vi "Phase III control screen.vi"() -> ()   [LabVIEW 2020]
uses:
  UI Message handler/User Event - Stop/User Event - Stop.lvlib
  UI Message handler/Message Queue/Message Queue.lvlib
  Globals/Phase III Globals.vi
  Controls/boolean ref.ctl
  Controls/Config.ctl
panel:
  out "Decerleration- LOX":bool
  out "Steady- LOX":bool
  out "Acceleration LOX":bool
  in  "Exit RT":bool
  in  "Check Prefire Purge Preparation Readiness 19":bool
  in  "Check Prefire Purge Preparation Readiness 18":bool
  in  "Check Prefire Purge Preparation Readiness 17":bool
  in  "Check Prefire Purge Preparation Readiness 16":bool
  in  "Check Prefire Purge Preparation Readiness 15":bool
  in  "Check Prefire Purge Preparation Readiness 14":bool
  in  "Check Prefire Purge Preparation Readiness 13":bool
  in  "Check Prefire Purge Preparation Readiness 12":bool
  in  "Check Prefire Purge Preparation Readiness 11":bool
  in  "Check Prefire Purge Preparation Readiness 10":bool
  in  "Check Prefire Purge Preparation Readiness 9":bool
  in  "Check Prefire Purge Preparation Readiness 8":bool
  in  "Check Prefire Purge Preparation Readiness 7":bool
  in  "Check Prefire Purge Preparation Readiness 6":bool
  out "PPSU":bool
  out "RUN ACKNOWLEDGE LOX":bool
  out "Shaft Rotational Direction":string
  out "Speed RPM -lox":dbl format="%#_g r/min"
  out "Frequency":dbl format="%#_g Hz"
  in  "SPEED                      l":dbl format="%#_g r/m"
  in  "RAMP DOWN      l":dbl format="%#_g S"
  in  "RAMP UP             l":dbl format="%#_g S"
  in  "SET FREQ             l":dbl format="%#_g Hz"
  out "RUN ACKNOWLEDGE Atf":bool
  out "Shaft Rotational Direction":string
  out "Speed RPM":dbl format="%#_g r/min"
  out "Frequency":dbl format="%#_g Hz"
  out "Terminal Power":dbl format="%#_g W"
  out "Terminal Current":dbl format="%#_g A"
  out "Terminal Voltage":dbl format="%#_g V"
  out "C_EPV_16 HSS":bool
  in  "C_EPV_16":bool
  out "N_EPV_202 HSS":bool
  in  "N_EPV_202":bool
  out "C_EPV_1352 HSS":bool
  in  "C_EPV_1352":bool
  out "C_EPV_18 HSS":bool
  in  "C_EPV_18":bool
  out "C_EPV_803 HSS":bool
  in  "C_EPV_803":bool
  out "N_EPV_141 HSS":bool
  in  "N_EPV_141":bool
  out "G_EPV_51 HSS":bool
  in  "G_EPV_51":bool
  out "N_EPV_61 HSS":bool
  in  "N_EPV_61":bool
  out "N_EPV_62b HSS":bool
  in  "N_EPV_62b":bool
  out "N_EPV_62a HSS":bool
  in  "N_EPV_62a":bool
  out "C_EPV_127 HSS":bool
  in  "C_EPV_127":bool
  out "C_EPV_123 HSS":bool
  in  "C_EPV_123":bool
  out "C_EPV_8 HSS":bool
  in  "C_EPV_8":bool
  out "C_EPV_7 HSS":bool
  in  "C_EPV_7":bool
  out "C_EPV_2 HSS":bool
  in  "C_EPV_2":bool
  out "N_EPV_75 HSS":bool
  in  "F_EPV_75":bool
  out "N_EPV_206 HSS":bool
  in  "N_EPV_206":bool
  out "N_EPV_203 HSS":bool
  in  "N_EPV_203":bool
  out "F_EPV_28 HSS":bool
  in  "F_EPV_28":bool
  out "N_EPV_142 HSS":bool
  in  "F_EPV_142":bool
  out "N_EPV_33 HSS":bool
  in  "N_EPV_ 33":bool
  out "N_EPV_69 HSS":bool
  in  "N_EPV_ 69":bool
  out "N_EPV_68 HSS":bool
  in  "N_EPV_68":bool
  out "F_EPV_41 HSS":bool
  in  "F_EPV_41":bool
  out "F_EPV_21 HSS":bool
  in  "F_EPV_21":bool
  out "F_EPV_132 HSS":bool
  in  "F_EPV_132":bool
  out "F_EPV_131 HSS":bool
  in  "F_EPV_131":bool
  out "F_EPV_136 HSS":bool
  in  "F_EPV_136":bool
  out "MS failure":bool
  out "Over power detection":bool
  out "Over current detection":bool
  out "over voltage detection":bool
  out "power failure status":bool
  out "Decerleration- ATF":bool
  out "Steady- ATF":bool
  out "Acceleration atf":bool
  out "LOG":bool
  out "TARGET":bool
  out "DR L":bool
  out "DR A":bool
  out "DO":bool
  out "DI":bool
  out "AO":bool
  out "AI":bool
  in  "ADC reset ATF":bool
  in  "MCU reset ATF":bool
  in  "Gate driver ATF":bool
  in  "Motor off ATF":bool
  in  "Motor On ATF":bool
  in  "Update drive ATF":bool
  in  "Adc reset lox":bool
  in  "MCU Reset -LOX":bool
  in  "Gate driver- LOX":bool
  in  "DC off":bool
  in  "DC on":bool
  in  "update ppsu":bool
  in  "Motor Off lox":bool
  in  "Motor On lox":bool
  in  "Update drive lox":bool
  in  "STOP LOG":bool
  in  "SPEED":dbl format="%#_g r/m"
  in  "RAMP DOWN":dbl format="%#_g S"
  in  "RAMP UP":dbl format="%#_g S"
  in  "SET FREQ":dbl format="%#_g Hz"
  in  "SET POWER":dbl format="%#_g W"
  in  "SET CURRENT":dbl format="%#_g A"
  in  "SET VOLTAGE":dbl format="%#_g V"
  in  "OPP(W)":dbl format="%#_g W"
  in  "OCP(A)":dbl format="%#_g A"
  in  "OVP(V)":dbl format="%#_g V"
  in  "Ms initialize":bool
  in  "Alarm ack":bool
  in  "Connect Drive Lox":bool
  in  "Connect Drive ATF":bool
  out "Time Stamp":timestamp format="%<%.3X>T"
  in  "Configure IP":bool
  in  "Datalog phase code":string(combo)
  in  "ABORT":bool
  in  "CONFIGURATION FILE":string(combo)
  in  "IP ADDRESS":string
  in  "HOLD UPDATE":bool
  in  "DAQ SETTING":bool
  in  "Connect ppsu":bool
  in  "Connect RT":bool
  in  "STOP DAQ":bool
  in  "EXIT":bool
  in  "START LOG":bool
  in  "START DAQ":bool
  # "VERSION NUMBER : 1.1"
  # "PHASE III"
  # "RELEASE DATE :03/05/24"
  # "Select the configuration file"
  # "Select the phase code"
  # "USER NAME :"
  # "SEQUENCE"
  # "ATF"
  # "LOX"
  # "ENGINE"
  # "EPV CONTROLS"
  # "EPV CONTROLS"
  # "EPV CONTROLS"
  # "Drive ATF Controls"
  # "Drive LOX Controls"
  # "PPSU"
  # "DRIVE ATF"
  # "DRIVE LOX"
  # "PPSU Controls"
  # "PPSU FEEDBACK PARAMETER"
  # "DRIVE ATF SET PARAMETER"
  # "Motor Rotational State"
  # "PPSU SET PARAMETER"
  # "DRIVE LOX SET PARAMETER"
  # "Motor Rotational State"
  # "PPSU FEEDBACK PARAMETER"
  # "DRIVE ATF FEEDBACK PARAMETER"
  # "DRIVE ATF FEEDBACK PARAMETER"
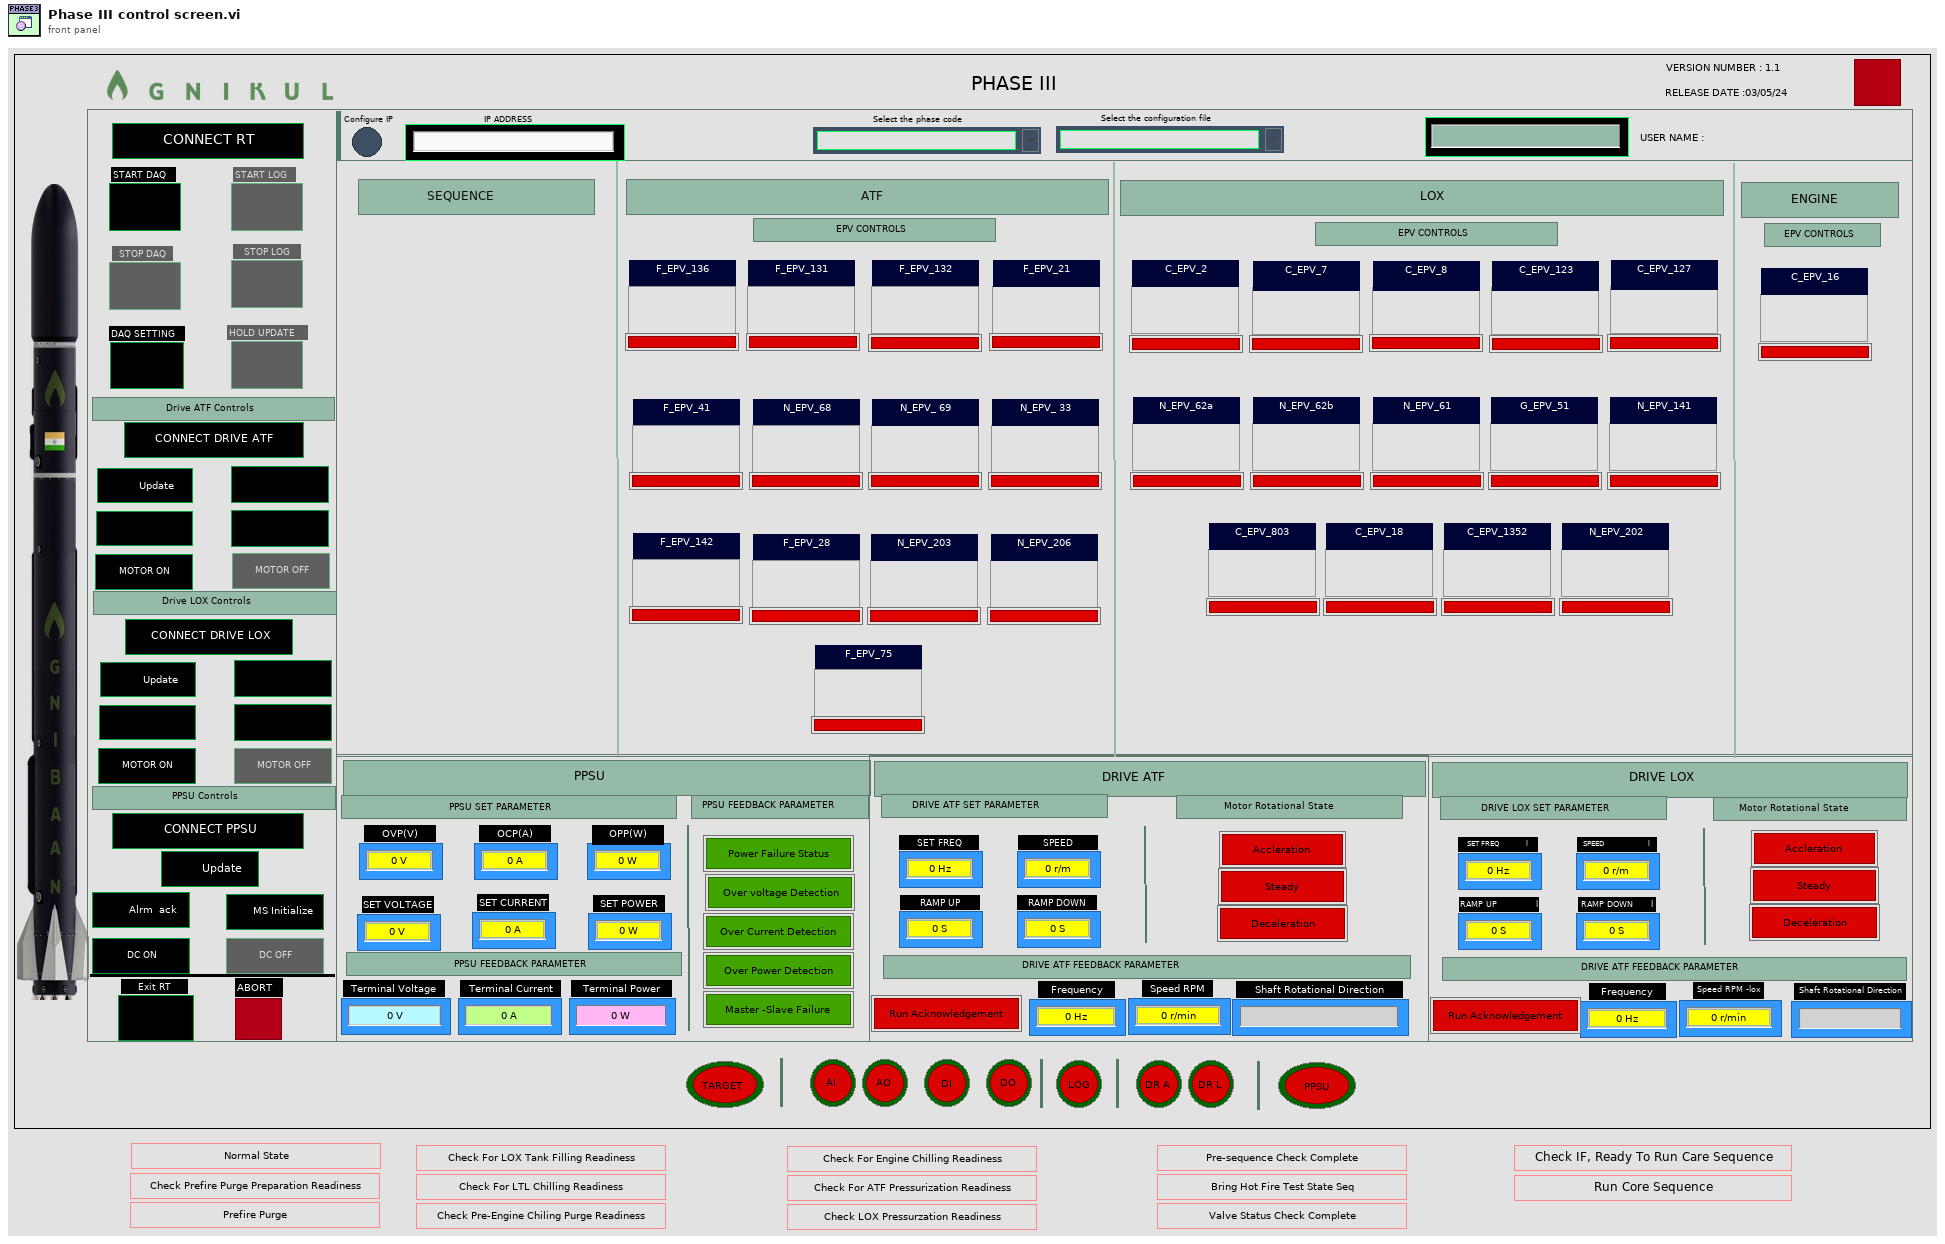
[diagram p1: front panel]
types:
  T1 = typedef "boolean ref.ctl" = cluster{"Connect RT":refnum<vi>, "START DAQ":refnum<vi>, "STOP DAQ":refnum<vi>, "DAQ SETTING":refnum<vi>, "START LOG":refnum<vi>, "STOP LOG":refnum<vi>, "Connect Drive ATF":refnum<vi>, "Update drive ATF":refnum<vi>, "Gate driver ATF":refnum<vi>, "Motor On ATF":refnum<vi>, "ADC reset ATF":refnum<vi>, "Gate driver ATF 2":refnum<vi>, "Motor off ATF":refnum<vi>, "MCU reset ATF":refnum<vi>, "Connect Drive Lox":refnum<vi>, "Update drive lox":refnum<vi>, "Gate driver- LOX":refnum<vi>, "Motor On lox":refnum<vi>, "Adc reset lox":refnum<vi>, "MCU Reset -LOX":refnum<vi>, "Motor Off lox":refnum<vi>, "Connect ppsu":refnum<vi>, "update ppsu":refnum<vi>, "DC on":refnum<vi>, "Alarm ack":refnum<vi>, "DC off":refnum<vi>, "Ms initialize":refnum<vi>, "Exit RT":refnum<vi>, "ABORT":refnum<vi>, "HOLD UPDATE":refnum<vi>}
  T2 = enum8{"Enabled", "Disabled", "Disabled and Grayed Out"}[]
  T3 = typedef "file folder ctl.ctl" = cluster{"Datalog path":path, "Configuration path":path, "Signal list path":path, "Sub vi's":path, "Authentication":path}
  T4 = typedef "Notifier ctl.ctl" = cluster{"Data":refnum<notifier>}
  T5 = typedef "Message Queue.lvlib/All Message Queues.ctl" = cluster{"UI":refnum<queue>, "NS ":refnum<queue>}
  T6 = typedef "Config.ctl" = cluster{"AO config":cluster{"Channel_Name":string, "Channel_Number":string, "Default_Value":dbl, "Units":string}[], "AI config":cluster{"Channel_Name":string, "Channel_Number":string, "Pre_Scale_min":dbl, "Pre_Scale_max":dbl, "Sensor_min":dbl, "Sensor_max":dbl, "Units":string}[], "DI config":cluster{"Channel_Name":string, "Channel_Number":string, "Default_Value":bool, "DI invert?":bool}[], "DO config":cluster{"Channel_Name":string, "Channel_Number":string, "Default_Value":bool, "DO invert?":bool}[], "TC config":cluster{"Channel_Name":string, "Channel_Number":string, "Pre_Scale_min":dbl, "Pre_Scale_max":dbl, "units":i32, " type":i32}[], "ACC config":cluster{"Channel_Name":string, "Channel_Number":string, "Pre_Scale_min":dbl, "Pre_Scale_max":dbl, "Terminal configuration":i32, "Sensitivity":dbl, "Sensitivity units":i32}[], "SG config":cluster{"Channel_Name":string, "Channel_Number":string, "Pre_Scale_min":dbl, "Pre_Scale_max":dbl}[], "Strain Gauge Settings":cluster{"poisson ratio":dbl, "nominal gage resistance":dbl, "gage factor":dbl}, "Bridge Settings":cluster{"voltage excitation value":dbl, "voltage excitation source":i32, "initial bridge voltage":dbl, "lead wire resistance":dbl, "strain configuration":i32}, "Sample Rate":cluster{"AI Sample Rate":dbl[], "AO Sample Rate":dbl[], "DI Sample Rate":dbl[], "TC Sample Rate":dbl[], "DO Sample Rate":dbl[], "SG Sample Rate":dbl[], "ACC Sample Rate":dbl[]}}
  T7 = enum16{"open", "replace", "create", "open or create", "replace or create", "replace or create with confirmation"}
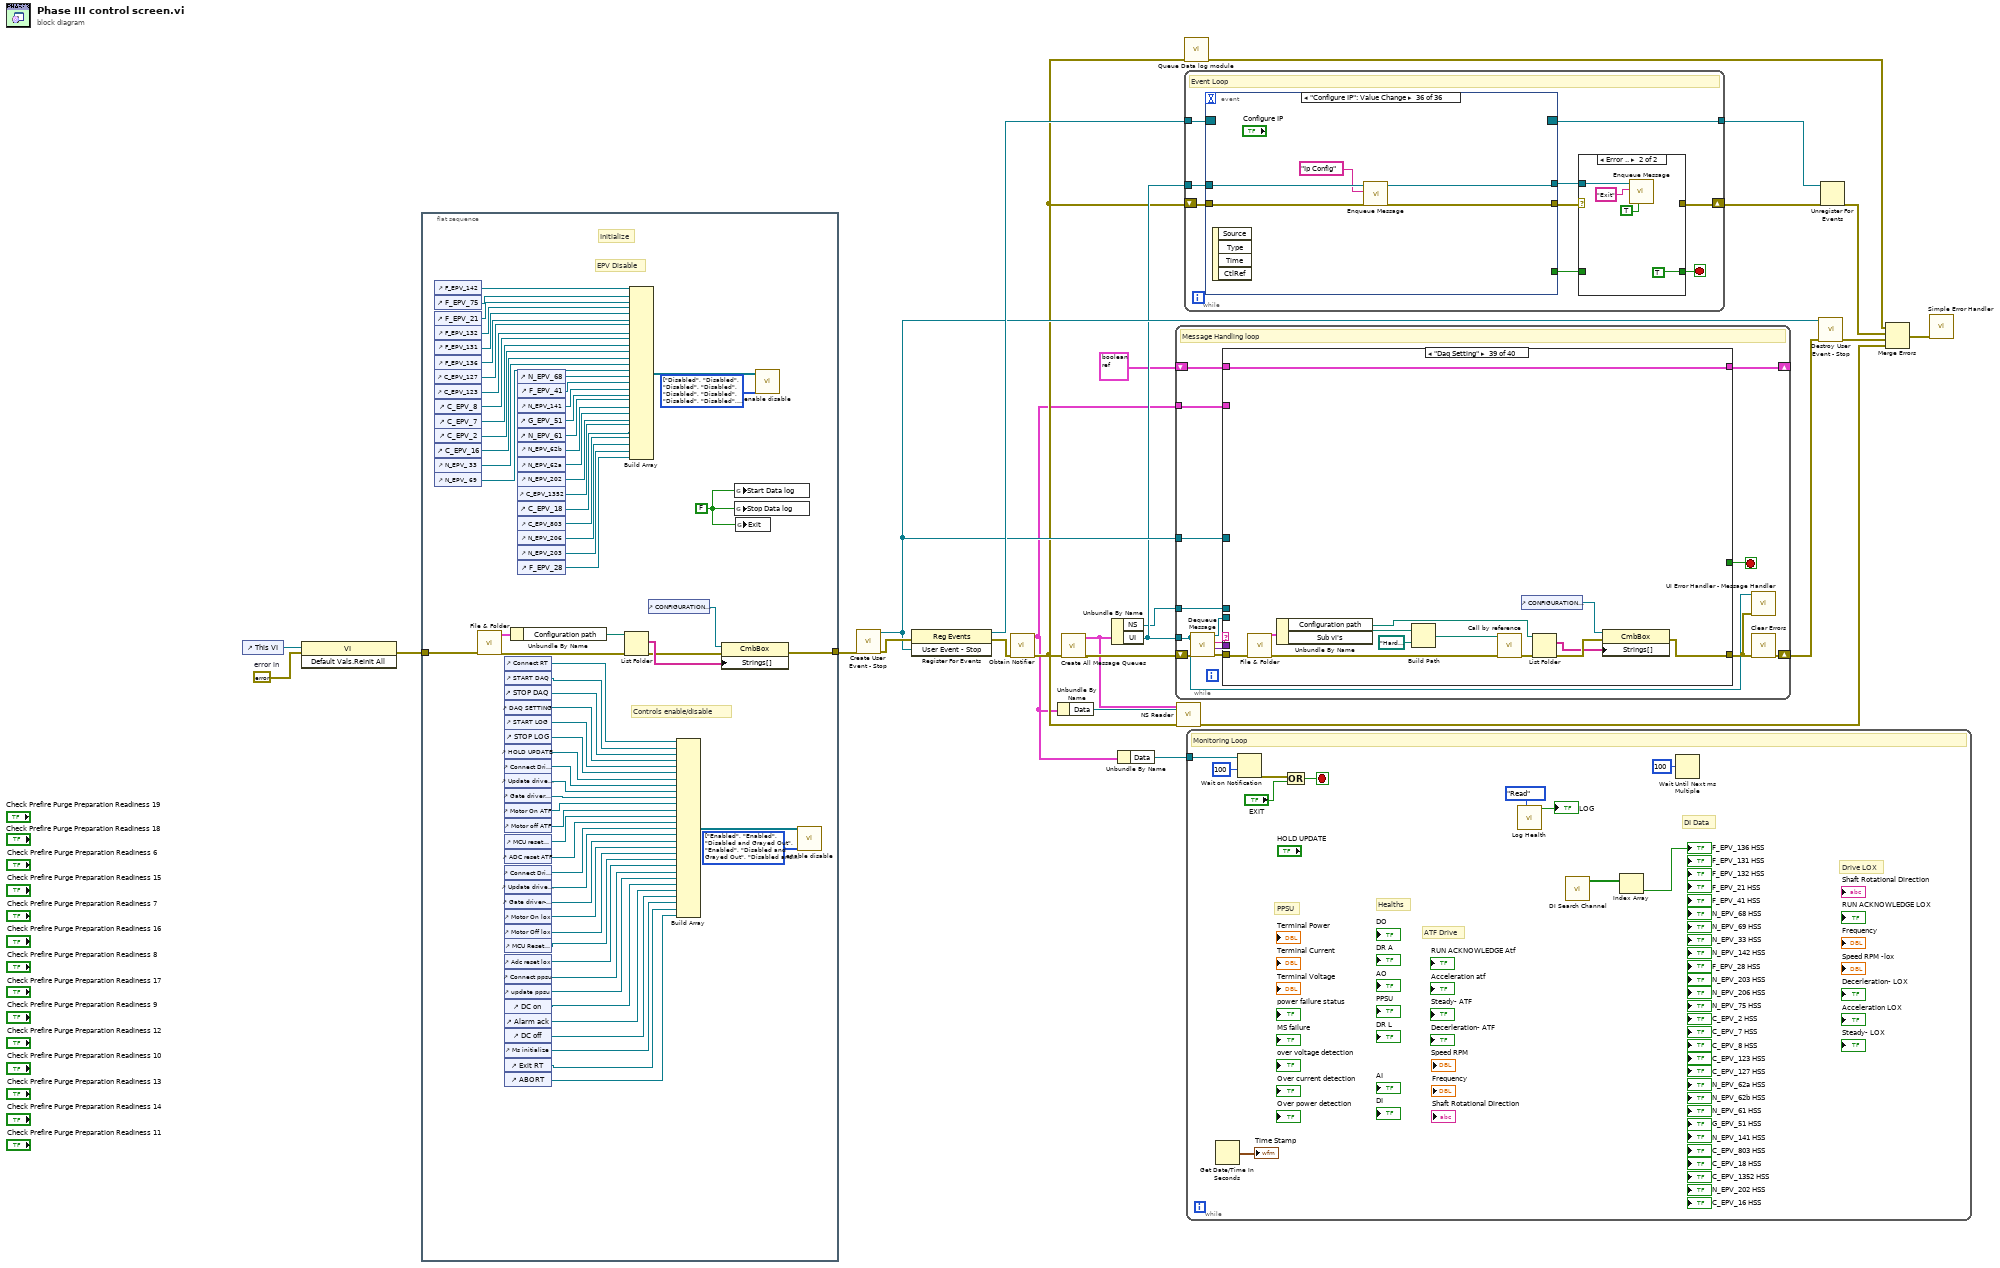
[diagram p0: block diagram]
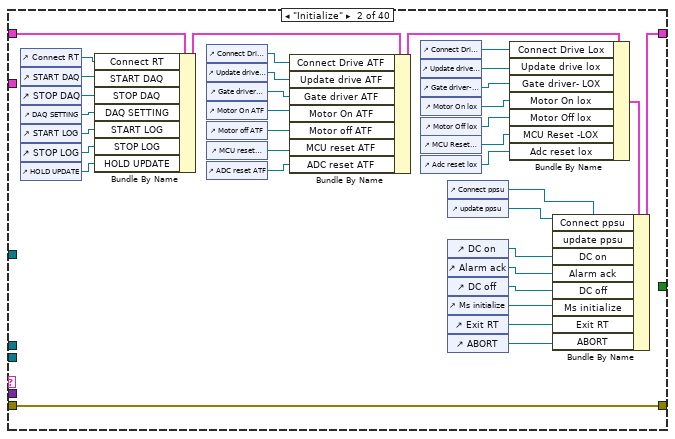
[diagram p3: hidden frame]
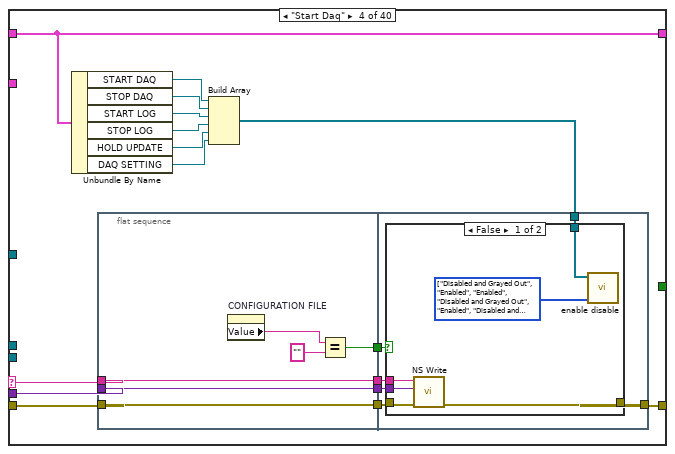
[diagram p5: hidden frame]
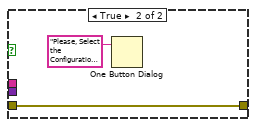
[diagram p6: hidden frame]
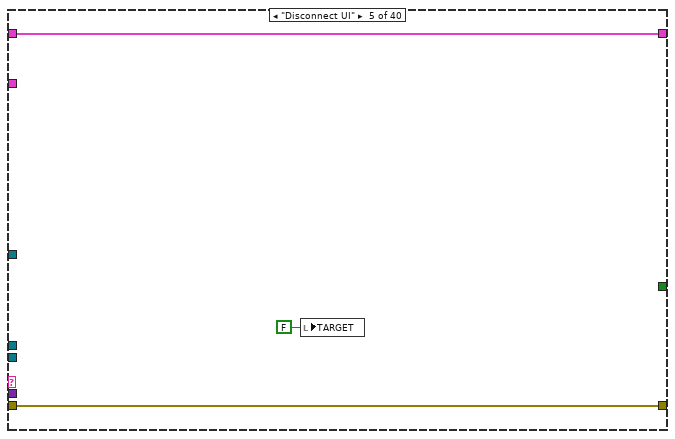
[diagram p7: hidden frame]
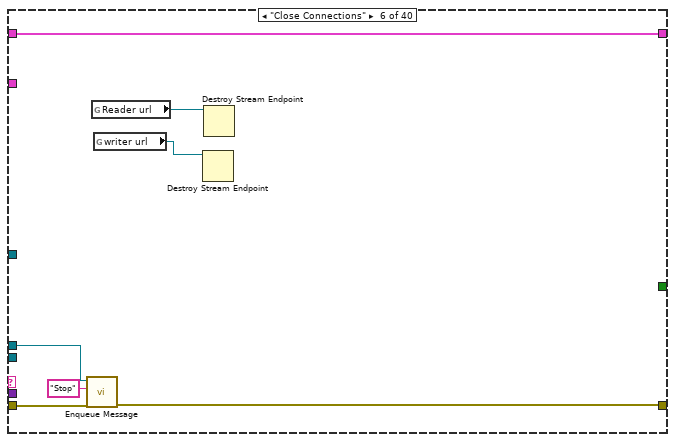
[diagram p8: hidden frame]
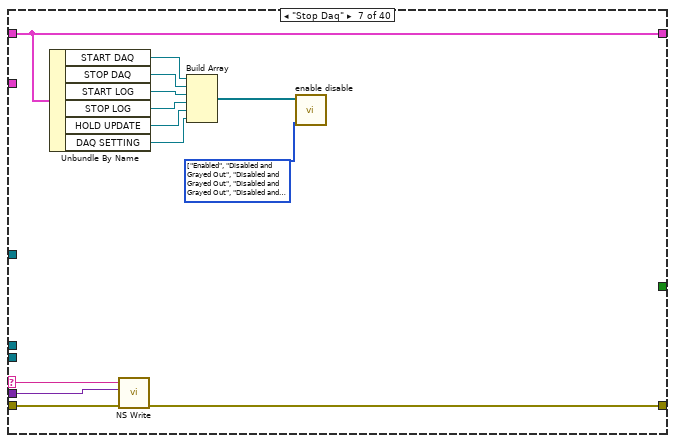
[diagram p9: hidden frame]
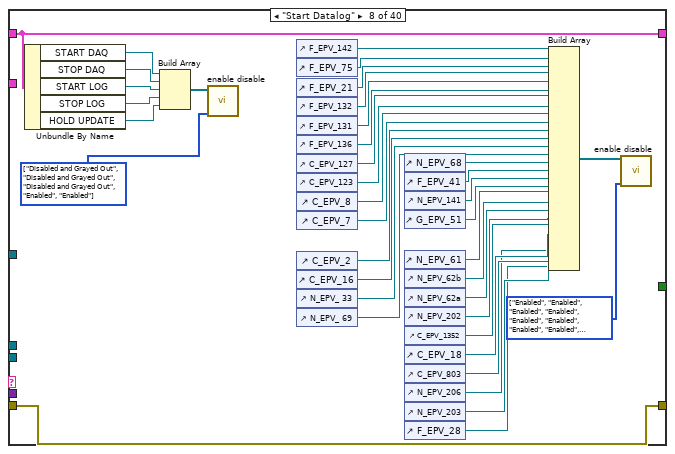
[diagram p10: hidden frame]
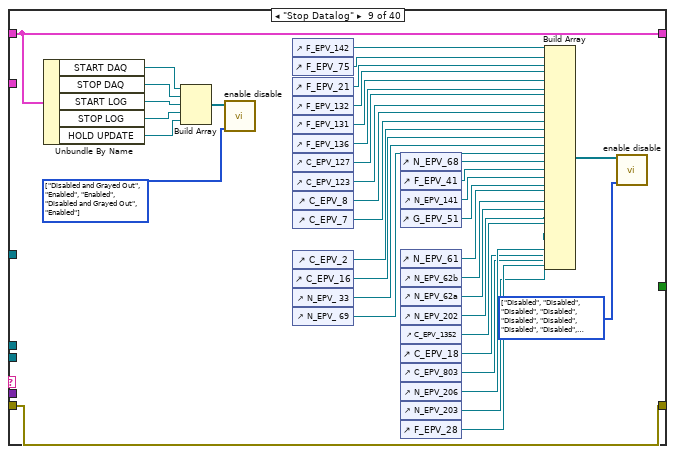
[diagram p11: hidden frame]
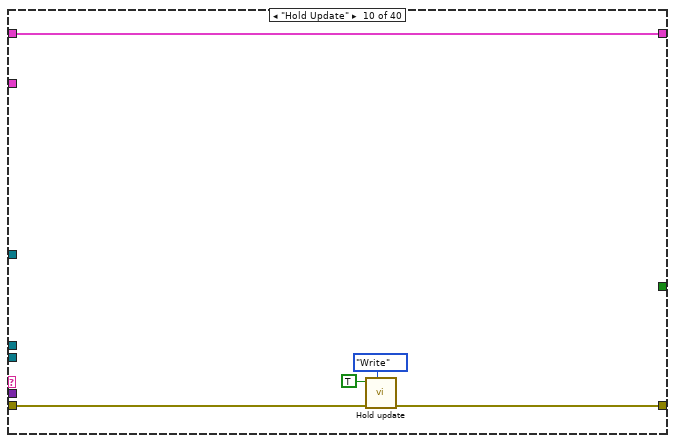
[diagram p12: hidden frame]
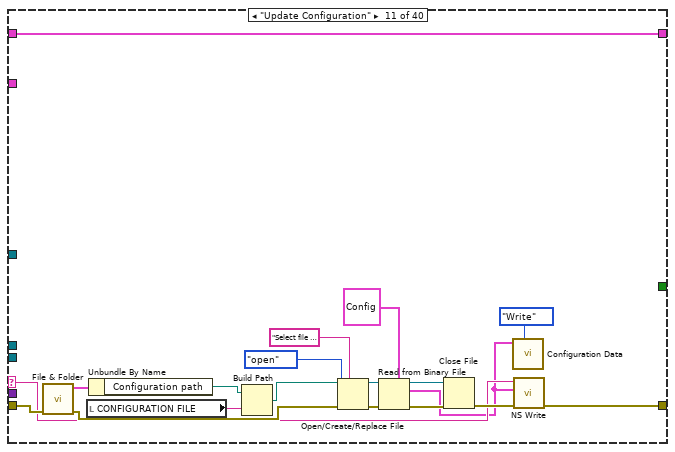
[diagram p13: hidden frame]
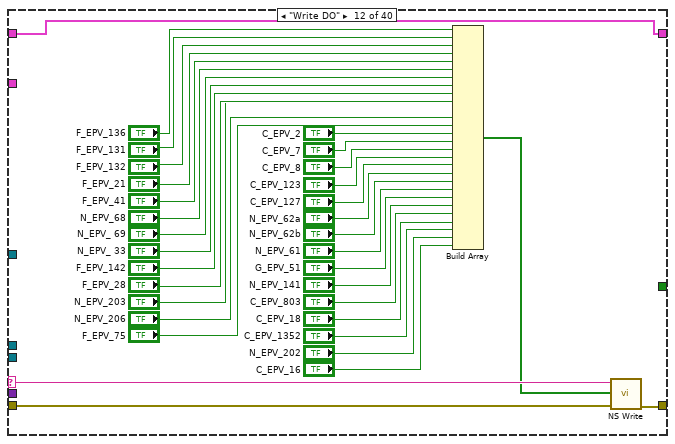
[diagram p14: hidden frame]
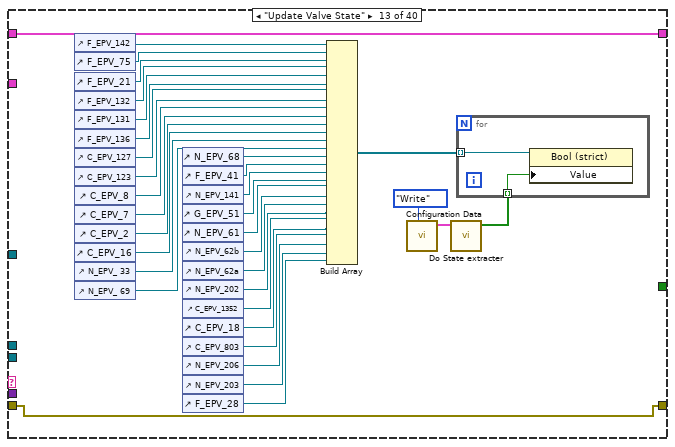
[diagram p15: hidden frame]
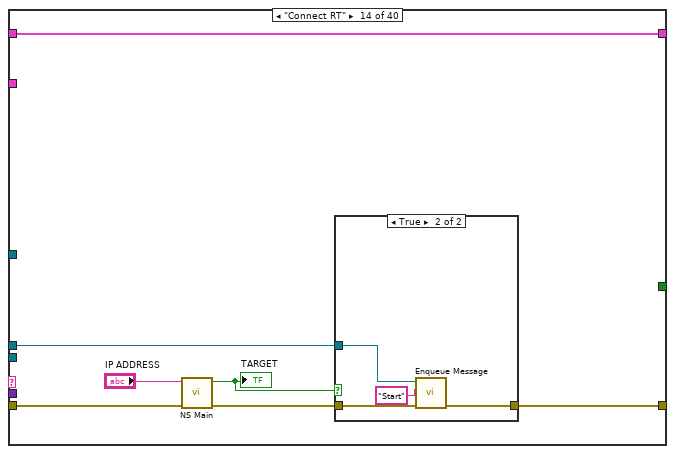
[diagram p16: hidden frame]
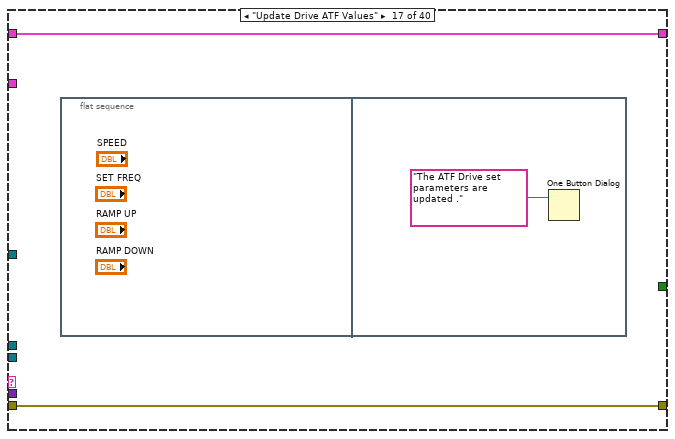
[diagram p20: hidden frame]
diagram:
  w2 = errorcluster {"status"=FALSE, "code"=0, "source"=""}  # error in
  n1 = control-ref of="This VI"() -> (w4:refnum<vi>)
  n2 = invoke class="VI" method="Default Vals.Reinit All"(reference=w4, error in=w2) -> (error out=w1:errorcluster)  [unwired: 1 in, 2 out]
  n3 = flat-sequence {
    tunnel: w1 -> [w31]
    tunnel: [w33] -> w16
    frame #0 {
      w34 = T2 [enum."Disabled", enum."Disabled", enum."Disabled", enum."Disabled", enum."Disabled", enum."Disabled", enum."Disabled", enum."Disabled", enum."Disabled", enum."Disabled", enum."Disabled", enum."Disabled", enum."Disabled", enum."Disabled", enum."Disabled", enum."Disabled", enum."Disabled", enum."Disabled", enum."Disabled", enum."Disabled", enum."Disabled", enum."Disabled", enum."Disabled", enum."Disabled", enum."Disabled", enum."Disabled", enum."Disabled", enum."Enabled", enum."Disabled"] items=["Enabled", "Disabled", "Disabled and Grayed Out"] ("Disabled")
      w65 = T2 [enum."Enabled", enum."Enabled", enum."Disabled and Grayed Out", enum."Enabled", enum."Disabled and Grayed Out", enum."Disabled and Grayed Out", enum."Disabled and Grayed Out", enum."Enabled", enum."Enabled", enum."Enabled", enum."Enabled", enum."Disabled and Grayed Out", enum."Enabled", enum."Enabled", enum."Enabled", enum."Enabled", enum."Enabled", enum."Enabled", enum."Disabled and Grayed Out", enum."Enabled", enum."Enabled", enum."Enabled", enum."Enabled", enum."Enabled", enum."Enabled", enum."Disabled and Grayed Out", enum."Enabled", enum."Enabled", enum."Enabled"] items=["Enabled", "Disabled", "Disabled and Grayed Out"] ("Disabled")
      w95 = FALSE ("Start Data log")
      # "Controls enable/disable"
      # "EPV Disable"
      # "Initialize"
      n4 = control-ref of="F_EPV_142"() -> (w35:refnum<vi>)
      n5 = control-ref of="F_EPV_75"() -> (w36:refnum<vi>)
      n6 = control-ref of="F_EPV_21"() -> (w37:refnum<vi>)
      n7 = control-ref of="F_EPV_132"() -> (w38:refnum<vi>)
      n8 = control-ref of="F_EPV_131"() -> (w39:refnum<vi>)
      n9 = control-ref of="F_EPV_136"() -> (w40:refnum<vi>)
      n10 = control-ref of="C_EPV_127"() -> (w41:refnum<vi>)
      n11 = control-ref of="C_EPV_123"() -> (w42:refnum<vi>)
      n12 = control-ref of="C_EPV_8"() -> (w43:refnum<vi>)
      n13 = control-ref of="C_EPV_7"() -> (w44:refnum<vi>)
      n14 = control-ref of="C_EPV_2"() -> (w45:refnum<vi>)
      n15 = control-ref of="C_EPV_16"() -> (w46:refnum<vi>)
      n16 = control-ref of="N_EPV_ 33"() -> (w47:refnum<vi>)
      n17 = control-ref of="N_EPV_ 69"() -> (w48:refnum<vi>)
      n18 = call "File & Folder.vi"("error in (no error)"=w31) -> ("error out"=w27:errorcluster, "File Output"=w30:T3)  [unwired: 9 in]
      n19 = control-ref of="Connect RT"() -> (w94:refnum<vi>)
      n20 = control-ref of="START DAQ"() -> (w93:refnum<vi>)
      n21 = control-ref of="STOP DAQ"() -> (w92:refnum<vi>)
      n22 = control-ref of="DAQ SETTING"() -> (w91:refnum<vi>)
      n23 = control-ref of="START LOG"() -> (w90:refnum<vi>)
      n24 = control-ref of="STOP LOG"() -> (w89:refnum<vi>)
      n25 = control-ref of="HOLD UPDATE"() -> (w88:refnum<vi>)
      n26 = control-ref of="Connect Drive ATF"() -> (w87:refnum<vi>)
      n27 = control-ref of="Update drive ATF"() -> (w86:refnum<vi>)
      n28 = control-ref of="Gate driver ATF"() -> (w85:refnum<vi>)
      n29 = control-ref of="Motor On ATF"() -> (w84:refnum<vi>)
      n30 = control-ref of="Motor off ATF"() -> (w83:refnum<vi>)
      n31 = control-ref of="MCU reset ATF"() -> (w82:refnum<vi>)
      n32 = control-ref of="ADC reset ATF"() -> (w81:refnum<vi>)
      n33 = control-ref of="Connect Drive Lox"() -> (w80:refnum<vi>)
      n34 = control-ref of="Update drive lox"() -> (w79:refnum<vi>)
      n35 = control-ref of="Gate driver- LOX"() -> (w78:refnum<vi>)
      n36 = control-ref of="Motor On lox"() -> (w77:refnum<vi>)
      n37 = control-ref of="Motor Off lox"() -> (w76:refnum<vi>)
      n38 = control-ref of="MCU Reset -LOX"() -> (w75:refnum<vi>)
      n39 = control-ref of="Adc reset lox"() -> (w74:refnum<vi>)
      n40 = control-ref of="Connect ppsu"() -> (w73:refnum<vi>)
      n41 = control-ref of="update ppsu"() -> (w72:refnum<vi>)
      n42 = control-ref of="DC on"() -> (w71:refnum<vi>)
      n43 = control-ref of="Alarm ack"() -> (w70:refnum<vi>)
      n44 = control-ref of="DC off"() -> (w69:refnum<vi>)
      n45 = control-ref of="Ms initialize"() -> (w68:refnum<vi>)
      n46 = control-ref of="Exit RT"() -> (w67:refnum<vi>)
      n47 = control-ref of="ABORT"() -> (w66:refnum<vi>)
      n48 = Unbundle By Name(w30) -> ("Configuration path"=w29:path)
      n49 = control-ref of="N_EPV_68"() -> (w49:refnum<vi>)
      n50 = control-ref of="F_EPV_41"() -> (w50:refnum<vi>)
      n51 = control-ref of="N_EPV_141"() -> (w51:refnum<vi>)
      n52 = control-ref of="G_EPV_51"() -> (w52:refnum<vi>)
      n53 = control-ref of="N_EPV_61"() -> (w53:refnum<vi>)
      n54 = control-ref of="N_EPV_62b"() -> (w54:refnum<vi>)
      n55 = control-ref of="N_EPV_62a"() -> (w55:refnum<vi>)
      n56 = control-ref of="N_EPV_202"() -> (w56:refnum<vi>)
      n57 = control-ref of="C_EPV_1352"() -> (w57:refnum<vi>)
      n58 = control-ref of="C_EPV_18"() -> (w58:refnum<vi>)
      n59 = control-ref of="C_EPV_803"() -> (w59:refnum<vi>)
      n60 = control-ref of="N_EPV_206"() -> (w60:refnum<vi>)
      n61 = control-ref of="N_EPV_203"() -> (w61:refnum<vi>)
      n62 = control-ref of="F_EPV_28"() -> (w62:refnum<vi>)
      n63 = List Folder(path=w29, error in=w27) -> (filenames=w28:string[], error out=w26:errorcluster)  [unwired: 2 in, 2 out]
      n64 = Build Array(w35, w36, w37, w38, w39, w40, w41, w42, w43, w44, w45, w46, w47, w48, w49, w50, w51, w52, w53, w54, w55, w56, w57, w58, w59, w60, w61, w62) -> (w63:refnum<vi>[])
      n65 = control-ref of="CONFIGURATION FILE"() -> (w32:refnum<vi>)
      n66 = Build Array(w94, w93, w92, w91, w90, w89, w88, w87, w86, w85, w84, w83, w82, w81, w80, w79, w78, w77, w76, w75, w74, w73, w72, w71, w70, w69, w68, w67, w66) -> (w64:refnum<vi>[])
      n67 = property class="CmbBox"(reference=w32, error in=w26, "Strings[]"=w28) -> (error out=w33:errorcluster)  [unwired: 1 out]
      n68 = global write "Phase III Globals.vi" "Start Data log"(w95) -> ()
      n69 = global write "Phase III Globals.vi" "Stop Data log"(w95) -> ()
      n70 = global write "Phase III Globals.vi" "Exit"(w95) -> ()
      n71 = call "enable disable.vi"("Disabled"=w34, "ref in"=w63) -> ()  [unwired: 10 in]
      n72 = call "enable disable.vi"("Disabled"=w65, "ref in"=w64) -> ()  [unwired: 10 in]
    }
  }
  n73 = call "Create User Event - Stop.vi"("error in (no error)"=w16) -> ("error out"=w22:errorcluster, "User Event - Stop"=w20:refnum<user-event>)  [unwired: 9 in]
  n74 = register-events(error in=w22, w20) -> (reference out=w25:refnum<event-registration>, error out=w15:errorcluster)  [unwired: 1 in]
  n75 = call "Obtain Notifier.vi"("error in"=w15) -> ("error out"=w8:errorcluster, "Notifier Out"=w5:T4)  [unwired: 9 in]
  n76 = Unbundle By Name(w5) -> ("Data"=w9:refnum<notifier>)
  n77 = call "Create All Message Queues.vi"("error in (no error)"=w8) -> ("error out"=w19:errorcluster, "Message Queues out"=w10:T5)  [unwired: 9 in]
  n78 = Unbundle By Name(w10) -> ("NS"=w6:refnum<queue>, "UI"=w18:refnum<queue>)
  n79 = Unbundle By Name(w5) -> ("Data"=w14:refnum<notifier>)
  n80 = while {
    shift-right: [w109] -> w13
    shift-left: w19 -> [w106]
    tunnel: w20 -> [w107]
    tunnel: w18 -> [w99]
    tunnel: w6 -> [w101]
    tunnel: w5 -> [w100]
    shift-right: [w96] -> _
    shift-left: T1 {"Connect RT"=refnum, "START DAQ"=refnum, "STOP DAQ"=refnum, "DAQ SETTING"=refnum, "START LOG"=refnum, "STOP LOG"=refnum, "Connect Drive ATF"=refnum, "Update drive ATF"=refnum, "Gate driver ATF"=refnum, "Motor On ATF"=refnum, "ADC reset ATF"=refnum, "Gate driver ATF 2"=refnum, "Motor off ATF"=refnum, "MCU reset ATF"=refnum, "Connect Drive Lox"=refnum, "Update drive lox"=refnum, "Gate driver- LOX"=refnum, "Motor On lox"=refnum, "Adc reset lox"=refnum, "MCU Reset -LOX"=refnum, "Motor Off lox"=refnum, "Connect ppsu"=refnum, "update ppsu"=refnum, "DC on"=refnum, "Alarm ack"=refnum, "DC off"=refnum, "Ms initialize"=refnum, "Exit RT"=refnum, "ABORT"=refnum, "HOLD UPDATE"=refnum} ("Cluster") -> [w97]
    stop <- w108 stop-if-true
    # "Message Handling loop"
    n81 = call "Dequeue Message.vi"("error in (no error)"=w106, "Message Queue"=w99) -> ("error out"=w105:errorcluster, "Message Data"=w102:variant, "Message"=w104:string, "dup Message Queue"=w103:refnum<queue>)  [unwired: 6 in]
    n82 = case shown="\"Daq Setting\"" w104 {
      selector: w104 -> [_ _ _ w163 _ _ w205 _ _ _ w293 w312 _ _ _ _ _ _ _ _ _ _ _ _ _ _ _ _ _ _ _ _ _ _ _ _ _ _ _ _]
      tunnel: w105 -> [w111 w146 w148 w162 w187 w190 w204 w208 w247 w289 w304 w314 w376 w385 w392 w394 w396 w399 w402 w404 w406 w416 w426 w428 w430 w432 w442 w452 w454 w463 w472 w474 w477 w479 w481 w486 w499 w504 w519 w521]
      tunnel: [w111 w146 w148 w161 w187 w188 w207 w208 w247 w288 w294 w313 w376 w380 w392 w394 w396 w399 w402 w404 w406 w416 w426 w428 w430 w432 w442 w452 w454 w463 w472 w474 w477 w479 w481 w493 w498 w502 w507 w521] -> w98
      tunnel: [_ _ _ _ _ _ _ _ _ _ _ _ _ _ _ _ _ _ _ _ _ _ _ _ _ _ _ _ _ _ _ _ _ _ _ TRUE ("EXIT") _ _ _ _] -> w108
      tunnel: w107 -> [_ _ _ _ _ _ _ _ _ _ _ _ _ _ _ _ _ _ _ _ _ _ _ _ _ _ _ _ _ _ _ _ _ _ _ w495 _ _ _ _]
      tunnel: w103 -> [_ _ _ _ _ _ _ _ _ _ _ _ _ _ _ _ _ _ _ _ _ _ _ _ _ _ _ _ _ _ _ _ _ _ _ w494 _ _ _ _]
      tunnel: w102 -> [_ _ _ w164 _ _ w206 _ _ _ _ _ _ _ _ _ _ _ _ _ _ _ _ _ _ _ _ _ _ _ _ _ _ _ _ _ _ _ _ _]
      tunnel: w101 -> [_ _ _ _ _ w189 _ _ _ _ _ _ _ w382 _ _ _ _ _ _ _ _ _ _ _ _ _ _ _ _ _ _ _ _ _ w484 _ _ _ _]
      tunnel: w100 -> [_ _ _ _ _ _ _ _ _ _ _ _ _ _ _ _ _ _ _ _ _ _ _ _ _ _ _ _ _ _ _ _ _ _ _ w491 _ _ _ _]
      tunnel: w97 -> [w110 w145 w147 w160 w185 w192 w196 w239 w279 w290 w309 w310 w375 w379 w391 w393 w395 w398 w401 w403 w405 w415 w418 w427 w429 w431 w441 w443 w453 w462 w464 w473 w476 w478 w480 w482 w501 w506 w513 w520]
      tunnel: [w110 w120 w147 w160 w185 w192 w196 w239 w279 w290 w309 w310 w375 w379 w391 w393 w395 w398 w401 w403 w405 w415 w418 w427 w429 w431 w441 w443 w453 w462 w464 w473 w476 w478 w480 w482 w501 w506 w513 w520] -> w96
      frame "Pole event", Default {
      }
      frame "Initialize" {
        n83 = control-ref of="Connect RT"() -> (w143:refnum<vi>)
        n84 = control-ref of="START DAQ"() -> (w142:refnum<vi>)
        n85 = control-ref of="STOP DAQ"() -> (w141:refnum<vi>)
        n86 = control-ref of="DAQ SETTING"() -> (w140:refnum<vi>)
        n87 = control-ref of="START LOG"() -> (w139:refnum<vi>)
        n88 = control-ref of="STOP LOG"() -> (w138:refnum<vi>)
        n89 = control-ref of="HOLD UPDATE"() -> (w137:refnum<vi>)
        n90 = Bundle By Name(cluster=w145, "Connect RT"=w143, "START DAQ"=w142, "STOP DAQ"=w141, "DAQ SETTING"=w140, "START LOG"=w139, "STOP LOG"=w138, "HOLD UPDATE"=w137) -> (w144:T1)
        n91 = control-ref of="Connect Drive ATF"() -> (w135:refnum<vi>)
        n92 = control-ref of="Update drive ATF"() -> (w134:refnum<vi>)
        n93 = control-ref of="Gate driver ATF"() -> (w133:refnum<vi>)
        n94 = control-ref of="Motor On ATF"() -> (w132:refnum<vi>)
        n95 = control-ref of="Motor off ATF"() -> (w131:refnum<vi>)
        n96 = control-ref of="MCU reset ATF"() -> (w130:refnum<vi>)
        n97 = control-ref of="ADC reset ATF"() -> (w129:refnum<vi>)
        n98 = Bundle By Name(cluster=w144, "Connect Drive ATF"=w135, "Update drive ATF"=w134, "Gate driver ATF"=w133, "Motor On ATF"=w132, "Motor off ATF"=w131, "MCU reset ATF"=w130, "ADC reset ATF"=w129) -> (w136:T1)
        n99 = control-ref of="Connect Drive Lox"() -> (w128:refnum<vi>)
        n100 = control-ref of="Update drive lox"() -> (w127:refnum<vi>)
        n101 = control-ref of="Gate driver- LOX"() -> (w126:refnum<vi>)
        n102 = control-ref of="Motor On lox"() -> (w125:refnum<vi>)
        n103 = control-ref of="Motor Off lox"() -> (w124:refnum<vi>)
        n104 = control-ref of="MCU Reset -LOX"() -> (w123:refnum<vi>)
        n105 = control-ref of="Adc reset lox"() -> (w122:refnum<vi>)
        n106 = control-ref of="Connect ppsu"() -> (w119:refnum<vi>)
        n107 = control-ref of="update ppsu"() -> (w118:refnum<vi>)
        n108 = control-ref of="DC on"() -> (w117:refnum<vi>)
        n109 = control-ref of="Alarm ack"() -> (w116:refnum<vi>)
        n110 = control-ref of="DC off"() -> (w115:refnum<vi>)
        n111 = control-ref of="Ms initialize"() -> (w114:refnum<vi>)
        n112 = control-ref of="Exit RT"() -> (w113:refnum<vi>)
        n113 = control-ref of="ABORT"() -> (w112:refnum<vi>)
        n114 = Bundle By Name(cluster=w136, "Connect Drive Lox"=w128, "Update drive lox"=w127, "Gate driver- LOX"=w126, "Motor On lox"=w125, "Motor Off lox"=w124, "MCU Reset -LOX"=w123, "Adc reset lox"=w122) -> (w121:T1)
        n115 = Bundle By Name(cluster=w121, "Connect ppsu"=w119, "update ppsu"=w118, "DC on"=w117, "Alarm ack"=w116, "DC off"=w115, "Ms initialize"=w114, "Exit RT"=w113, "ABORT"=w112) -> (w120:T1)
      }
      frame "Ip Config" {
      }
      frame "Start Daq" {
        n116 = Unbundle By Name(w160) -> ("START DAQ"=w159:refnum<vi>, "STOP DAQ"=w158:refnum<vi>, "START LOG"=w157:refnum<vi>, "STOP LOG"=w156:refnum<vi>, "HOLD UPDATE"=w155:refnum<vi>, "DAQ SETTING"=w154:refnum<vi>)
        n117 = flat-sequence {
          tunnel: w162 -> [w168]
          tunnel: w163 -> [w169]
          tunnel: w164 -> [w170]
          tunnel: [w170] -> w153
          tunnel: [w169] -> w152
          tunnel: [w168] -> w151
          tunnel: [w165] -> w150
          tunnel: [w173] -> w161
          tunnel: w153 -> [w176]
          tunnel: w152 -> [w175]
          tunnel: w151 -> [w174]
          tunnel: w150 -> [w172]
          tunnel: w149 -> [w171]
          frame #0 {
            n118 = property on="CONFIGURATION FILE" class="CmbBox"() -> ("Value"=w167:string)  [unwired: 2 in, 2 out]
            n119 = Equal?(x=w167, y="") -> (x = y?=w165:bool)
          }
          frame #1 {
            n120 = case shown="False" w172 {
              tunnel: w176 -> [w182 _]
              tunnel: w175 -> [w181 _]
              tunnel: w174 -> [w180 w184]
              tunnel: [w179 w184] -> w173
              tunnel: w171 -> [w178 _]
              frame False {
                w177 = T2 [enum."Disabled and Grayed Out", enum."Enabled", enum."Enabled", enum."Disabled and Grayed Out", enum."Enabled", enum."Disabled and Grayed Out"] items=["Enabled", "Disabled", "Disabled and Grayed Out"] ("Disabled")
                n121 = call "NS Write.vi"("error in"=w180, "Data"=w182, "Message"=w181) -> ("error out"=w179:errorcluster)  [unwired: 8 in]
                n122 = call "enable disable.vi"("Disabled"=w177, "ref in"=w178) -> ()  [unwired: 10 in]
              }
              frame True {
                n123 = One Button Dialog(message="Please, Select the Configuration File !!") -> ()  [unwired: 1 in, 1 out]
              }
            }
          }
        }
        n124 = Build Array(w159, w158, w157, w156, w155, w154) -> (w149:refnum<vi>[])
      }
      frame "Disconnect UI" {
        n125 = local write "TARGET"(FALSE ("TARGET")) -> ()
      }
      frame "Close Connections" {
        n126 = call "Enqueue Message.vi"("error in (no error)"=w190, "Message"="Stop", "Message Queue"=w189) -> ("error out"=w188:errorcluster)  [unwired: 7 in, 1 out]
        n127 = global read "Phase III Globals.vi" "Reader url"() -> (w194:refnum<k21>)
        n128 = global read "Phase III Globals.vi" "writer url"() -> (w193:refnum<k21>)
        n129 = Destroy Stream Endpoint(11:w193) -> ()  [unwired: 1 in, 1 out]
        n130 = Destroy Stream Endpoint(11:w194) -> ()  [unwired: 1 in, 1 out]
      }
      frame "Stop Daq" {
        w197 = T2 [enum."Enabled", enum."Disabled and Grayed Out", enum."Disabled and Grayed Out", enum."Disabled and Grayed Out", enum."Disabled and Grayed Out", enum."Enabled"] items=["Enabled", "Disabled", "Disabled and Grayed Out"] ("Disabled")
        n131 = Unbundle By Name(w196) -> ("START DAQ"=w203:refnum<vi>, "STOP DAQ"=w202:refnum<vi>, "START LOG"=w201:refnum<vi>, "STOP LOG"=w200:refnum<vi>, "HOLD UPDATE"=w198:refnum<vi>, "DAQ SETTING"=w195:refnum<vi>)
        n132 = call "NS Write.vi"("error in"=w204, "Data"=w206, "Message"=w205) -> ("error out"=w207:errorcluster)  [unwired: 8 in]
        n133 = Build Array(w203, w202, w201, w200, w198, w195) -> (w199:refnum<vi>[])
        n134 = call "enable disable.vi"("Disabled"=w197, "ref in"=w199) -> ()  [unwired: 10 in]
      }
      frame "Start Datalog" {
        w209 = T2 [enum."Enabled", enum."Enabled", enum."Enabled", enum."Enabled", enum."Enabled", enum."Enabled", enum."Enabled", enum."Enabled", enum."Enabled", enum."Enabled", enum."Enabled", enum."Enabled", enum."Enabled", enum."Enabled", enum."Enabled", enum."Enabled", enum."Enabled", enum."Enabled", enum."Enabled", enum."Enabled", enum."Enabled", enum."Enabled", enum."Enabled", enum."Enabled", enum."Enabled", enum."Enabled", enum."Enabled", enum."Enabled", enum."Enabled"] items=["Enabled", "Disabled", "Disabled and Grayed Out"] ("Disabled")
        w240 = T2 [enum."Disabled and Grayed Out", enum."Disabled and Grayed Out", enum."Disabled and Grayed Out", enum."Enabled", enum."Enabled"] items=["Enabled", "Disabled", "Disabled and Grayed Out"] ("Disabled")
        n135 = Unbundle By Name(w239) -> ("START DAQ"=w246:refnum<vi>, "STOP DAQ"=w245:refnum<vi>, "START LOG"=w244:refnum<vi>, "STOP LOG"=w243:refnum<vi>, "HOLD UPDATE"=w241:refnum<vi>)
        n136 = Build Array(w246, w245, w244, w243, w241) -> (w242:refnum<vi>[])
        n137 = call "enable disable.vi"("Disabled"=w240, "ref in"=w242) -> ()  [unwired: 10 in]
        n138 = control-ref of="F_EPV_142"() -> (w238:refnum<vi>)
        n139 = control-ref of="F_EPV_75"() -> (w237:refnum<vi>)
        n140 = control-ref of="F_EPV_21"() -> (w236:refnum<vi>)
        n141 = control-ref of="F_EPV_132"() -> (w235:refnum<vi>)
        n142 = control-ref of="F_EPV_131"() -> (w234:refnum<vi>)
        n143 = control-ref of="F_EPV_136"() -> (w233:refnum<vi>)
        n144 = control-ref of="C_EPV_127"() -> (w232:refnum<vi>)
        n145 = control-ref of="C_EPV_123"() -> (w231:refnum<vi>)
        n146 = control-ref of="C_EPV_8"() -> (w230:refnum<vi>)
        n147 = control-ref of="C_EPV_7"() -> (w229:refnum<vi>)
        n148 = control-ref of="C_EPV_2"() -> (w228:refnum<vi>)
        n149 = control-ref of="C_EPV_16"() -> (w227:refnum<vi>)
        n150 = control-ref of="N_EPV_ 33"() -> (w226:refnum<vi>)
        n151 = control-ref of="N_EPV_ 69"() -> (w225:refnum<vi>)
        n152 = control-ref of="N_EPV_68"() -> (w224:refnum<vi>)
        n153 = control-ref of="F_EPV_41"() -> (w223:refnum<vi>)
        n154 = control-ref of="N_EPV_141"() -> (w222:refnum<vi>)
        n155 = control-ref of="G_EPV_51"() -> (w221:refnum<vi>)
        n156 = control-ref of="N_EPV_61"() -> (w220:refnum<vi>)
        n157 = control-ref of="N_EPV_62b"() -> (w219:refnum<vi>)
        n158 = control-ref of="N_EPV_62a"() -> (w218:refnum<vi>)
        n159 = control-ref of="N_EPV_202"() -> (w217:refnum<vi>)
        n160 = control-ref of="C_EPV_1352"() -> (w216:refnum<vi>)
        n161 = control-ref of="C_EPV_18"() -> (w215:refnum<vi>)
        n162 = control-ref of="C_EPV_803"() -> (w214:refnum<vi>)
        n163 = control-ref of="N_EPV_206"() -> (w213:refnum<vi>)
        n164 = control-ref of="N_EPV_203"() -> (w212:refnum<vi>)
        n165 = control-ref of="F_EPV_28"() -> (w211:refnum<vi>)
        n166 = Build Array(w238, w237, w236, w235, w234, w233, w232, w231, w230, w229, w228, w227, w226, w225, w224, w223, w222, w221, w220, w219, w218, w217, w216, w215, w214, w213, w212, w211) -> (w210:refnum<vi>[])
        n167 = call "enable disable.vi"("Disabled"=w209, "ref in"=w210) -> ()  [unwired: 10 in]
      }
      frame "Stop Datalog" {
        w248 = T2 [enum."Disabled", enum."Disabled", enum."Disabled", enum."Disabled", enum."Disabled", enum."Disabled", enum."Disabled", enum."Disabled", enum."Disabled", enum."Disabled", enum."Disabled", enum."Disabled", enum."Disabled", enum."Disabled", enum."Disabled", enum."Disabled", enum."Disabled", enum."Disabled", enum."Disabled", enum."Disabled", enum."Disabled", enum."Disabled", enum."Disabled", enum."Disabled", enum."Disabled", enum."Disabled", enum."Disabled", enum."Enabled", enum."Disabled"] items=["Enabled", "Disabled", "Disabled and Grayed Out"] ("Disabled")
        w280 = T2 [enum."Disabled and Grayed Out", enum."Enabled", enum."Enabled", enum."Disabled and Grayed Out", enum."Enabled"] items=["Enabled", "Disabled", "Disabled and Grayed Out"] ("Disabled")
        n168 = Unbundle By Name(w279) -> ("START DAQ"=w278:refnum<vi>, "STOP DAQ"=w285:refnum<vi>, "START LOG"=w284:refnum<vi>, "STOP LOG"=w283:refnum<vi>, "HOLD UPDATE"=w281:refnum<vi>)
        n169 = Build Array(w278, w285, w284, w283, w281) -> (w282:refnum<vi>[])
        n170 = call "enable disable.vi"("Disabled"=w280, "ref in"=w282) -> ()  [unwired: 10 in]
        n171 = control-ref of="F_EPV_142"() -> (w249:refnum<vi>)
        n172 = control-ref of="F_EPV_75"() -> (w250:refnum<vi>)
        n173 = control-ref of="F_EPV_21"() -> (w251:refnum<vi>)
        n174 = control-ref of="F_EPV_132"() -> (w252:refnum<vi>)
        n175 = control-ref of="F_EPV_131"() -> (w253:refnum<vi>)
        n176 = control-ref of="F_EPV_136"() -> (w254:refnum<vi>)
        n177 = control-ref of="C_EPV_127"() -> (w255:refnum<vi>)
        n178 = control-ref of="C_EPV_123"() -> (w256:refnum<vi>)
        n179 = control-ref of="C_EPV_8"() -> (w257:refnum<vi>)
        n180 = control-ref of="C_EPV_7"() -> (w258:refnum<vi>)
        n181 = control-ref of="C_EPV_2"() -> (w259:refnum<vi>)
        n182 = control-ref of="C_EPV_16"() -> (w260:refnum<vi>)
        n183 = control-ref of="N_EPV_ 33"() -> (w261:refnum<vi>)
        n184 = control-ref of="N_EPV_ 69"() -> (w262:refnum<vi>)
        n185 = control-ref of="N_EPV_68"() -> (w263:refnum<vi>)
        n186 = control-ref of="F_EPV_41"() -> (w264:refnum<vi>)
        n187 = control-ref of="N_EPV_141"() -> (w265:refnum<vi>)
        n188 = control-ref of="G_EPV_51"() -> (w266:refnum<vi>)
        n189 = control-ref of="N_EPV_61"() -> (w267:refnum<vi>)
        n190 = control-ref of="N_EPV_62b"() -> (w268:refnum<vi>)
        n191 = control-ref of="N_EPV_62a"() -> (w269:refnum<vi>)
        n192 = control-ref of="N_EPV_202"() -> (w270:refnum<vi>)
        n193 = control-ref of="C_EPV_1352"() -> (w271:refnum<vi>)
        n194 = control-ref of="C_EPV_18"() -> (w272:refnum<vi>)
        n195 = control-ref of="C_EPV_803"() -> (w273:refnum<vi>)
        n196 = control-ref of="N_EPV_206"() -> (w274:refnum<vi>)
        n197 = control-ref of="N_EPV_203"() -> (w275:refnum<vi>)
        n198 = control-ref of="F_EPV_28"() -> (w276:refnum<vi>)
        n199 = Build Array(w249, w250, w251, w252, w253, w254, w255, w256, w257, w258, w259, w260, w261, w262, w263, w264, w265, w266, w267, w268, w269, w270, w271, w272, w273, w274, w275, w276) -> (w277:refnum<vi>[])
        n200 = call "enable disable.vi"("Disabled"=w248, "ref in"=w277) -> ()  [unwired: 10 in]
      }
      frame "Hold Update" {
        n201 = call "Hold update .vi"("Enum"=enum16{"Read", "Write"}."Write", "error in (no error)"=w289, "In"=TRUE) -> ("error out"=w288:errorcluster)  [unwired: 7 in, 1 out]
      }
      frame "Update Configuration" {
        n202 = call "File & Folder.vi"("error in (no error)"=w304) -> ("error out"=w299:errorcluster, "File Output"=w303:T3)  [unwired: 9 in]
        n203 = local read "CONFIGURATION FILE"() -> (w301:string)
        n204 = Unbundle By Name(w303) -> ("Configuration path"=w302:path)
        n205 = Build Path(base path=w302, name or relative path=w301) -> (appended path=w300:path)
        n206 = Open/Create/Replace File(file path (use dialog)=w300, error in=w299, prompt="Select file to load", operation (0:open)=T7."open") -> (refnum out=w307:refnum<file>, error out=w298:errorcluster)  [unwired: 2 in, 1 out]
        n207 = Read from Binary File(5:T6 {"AO config"=[], "AI config"=[], "DI config"=[], "DO config"=[], "TC config"=[{"Channel_Name"="", "Channel_Number"="", "Pre_Scale_min"=0.0, "Pre_Scale_max"=0.0, "units"=4, " type"=7}], "ACC config"=[], "SG config"=[], "Strain Gauge Settings"={"poisson ratio"=0.3, "nominal gage resistance"=120.0, "gage factor"=2.08}, "Bridge Settings"={"voltage excitation value"=3.3, "voltage excitation source"=10200, "initial bridge voltage"=0.0, "lead wire resistance"=1.7, "strain configuration"=10271}, "Sample Rate"={"AI Sample Rate"=[], "AO Sample Rate"=[], "DI Sample Rate"=[], "TC Sample Rate"=[], "DO Sample Rate"=[], "SG Sample Rate"=[], "ACC Sample Rate"=[]}} ("Data"), 8:w298, 11:w307) -> (0:w297:errorcluster, 2:w291:T6, 3:w308:refnum<file>)  [unwired: 3 in, 1 out]
        n208 = Close File(refnum=w308, error in=w297) -> (error out=w295:errorcluster)  [unwired: 1 out]
        n209 = call "Configuration Data.vi"("Enum"=enum16{"Read", "Write"}."Write", "data"=w291) -> ()  [unwired: 8 in, 2 out]
        n210 = call "NS Write.vi"("error in"=w295, "Data"=w291, "Message"=w293) -> ("error out"=w294:errorcluster)  [unwired: 8 in]
      }
      frame "Write DO" {
        n211 = Build Array("F_EPV_136", "F_EPV_131", "F_EPV_132", "F_EPV_21", "F_EPV_41", "N_EPV_68", "N_EPV_ 69", "N_EPV_ 33", "F_EPV_142", "F_EPV_28", "N_EPV_203", "N_EPV_206", "F_EPV_75", "C_EPV_2", "C_EPV_7", "C_EPV_8", "C_EPV_123", "C_EPV_127", "N_EPV_62a", "N_EPV_62b", "N_EPV_61", "G_EPV_51", "N_EPV_141", "C_EPV_803", "C_EPV_18", "C_EPV_1352", "N_EPV_202", "C_EPV_16") -> (w311:bool[])
        n212 = call "NS Write.vi"("error in"=w314, "Data"=w311, "Message"=w312) -> ("error out"=w313:errorcluster)  [unwired: 8 in]
      }
      frame "Update Valve State" {
        n213 = control-ref of="F_EPV_142"() -> (w343:refnum<vi>)
        n214 = control-ref of="F_EPV_75"() -> (w371:refnum<vi>)
        n215 = control-ref of="F_EPV_21"() -> (w370:refnum<vi>)
        n216 = control-ref of="F_EPV_132"() -> (w369:refnum<vi>)
        n217 = control-ref of="F_EPV_131"() -> (w368:refnum<vi>)
        n218 = control-ref of="F_EPV_136"() -> (w367:refnum<vi>)
        n219 = control-ref of="C_EPV_127"() -> (w366:refnum<vi>)
        n220 = control-ref of="C_EPV_123"() -> (w365:refnum<vi>)
        n221 = control-ref of="C_EPV_8"() -> (w364:refnum<vi>)
        n222 = control-ref of="C_EPV_7"() -> (w363:refnum<vi>)
        n223 = control-ref of="C_EPV_2"() -> (w362:refnum<vi>)
        n224 = control-ref of="C_EPV_16"() -> (w361:refnum<vi>)
        n225 = control-ref of="N_EPV_ 33"() -> (w360:refnum<vi>)
        n226 = control-ref of="N_EPV_ 69"() -> (w359:refnum<vi>)
        n227 = control-ref of="N_EPV_68"() -> (w358:refnum<vi>)
        n228 = control-ref of="F_EPV_41"() -> (w357:refnum<vi>)
        n229 = control-ref of="N_EPV_141"() -> (w356:refnum<vi>)
        n230 = control-ref of="G_EPV_51"() -> (w355:refnum<vi>)
        n231 = control-ref of="N_EPV_61"() -> (w354:refnum<vi>)
        n232 = control-ref of="N_EPV_62b"() -> (w353:refnum<vi>)
        n233 = control-ref of="N_EPV_62a"() -> (w352:refnum<vi>)
        n234 = control-ref of="N_EPV_202"() -> (w351:refnum<vi>)
        n235 = control-ref of="C_EPV_1352"() -> (w350:refnum<vi>)
        n236 = control-ref of="C_EPV_18"() -> (w349:refnum<vi>)
        n237 = control-ref of="C_EPV_803"() -> (w348:refnum<vi>)
        n238 = control-ref of="N_EPV_206"() -> (w347:refnum<vi>)
        n239 = control-ref of="N_EPV_203"() -> (w346:refnum<vi>)
        n240 = control-ref of="F_EPV_28"() -> (w345:refnum<vi>)
        n241 = Build Array(w343, w371, w370, w369, w368, w367, w366, w365, w364, w363, w362, w361, w360, w359, w358, w357, w356, w355, w354, w353, w352, w351, w350, w349, w348, w347, w346, w345) -> (w344:refnum<vi>[])
        n242 = call "Configuration Data.vi"("Enum"=enum16{"Read", "Write"}."Write") -> ("data 2"=w373:T6)  [unwired: 9 in, 1 out]
        n243 = call "Do State extracter.vi"("input cluster"=w373) -> ("Do State"=w372:bool[])  [unwired: 10 in]
        n244 = for {
          tunnel: w372 -> [w378] mode=indexing
          tunnel: w344 -> [w377] mode=indexing
          n245 = property class="Bool (strict)"(reference=w377, "Value"=w378) -> ()  [unwired: 1 in, 2 out]
        }
      }
      frame "Connect RT" {
        n246 = call "NS Main.vi"("error in (no error)"=w385, "Ip Address"="IP ADDRESS") -> ("error out"=w381:errorcluster, "Connected  ?"=w383:bool)  [unwired: 8 in]
        "TARGET" <- w383
        n247 = case shown="True" w383 {
          tunnel: w382 -> [_ w389]
          tunnel: w381 -> [w386 w388]
          tunnel: [w386 w387] -> w380
          frame False {
          }
          frame True {
            n248 = call "Enqueue Message.vi"("error in (no error)"=w388, "Message"="Start", "Message Queue"=w389) -> ("error out"=w387:errorcluster)  [unwired: 7 in, 1 out]
          }
        }
      }
      frame "Connect Drive ATF" {
      }
      frame "Connect Drive LOX" {
      }
      frame "Update Drive ATF Values" {
        n249 = flat-sequence {
          frame #0 {
          }
          frame #1 {
            n250 = One Button Dialog(message="The ATF Drive set parameters are updated .") -> ()  [unwired: 1 in, 1 out]
          }
        }
      }
      frame "Update Drive LOX Values" {
        n251 = flat-sequence {
          frame #0 {
          }
          frame #1 {
            n252 = One Button Dialog(message="The LOX Drive set parameters are updated .") -> ()  [unwired: 1 in, 1 out]
          }
        }
      }
      frame "Gate Driver Power ATF" {
      }
      frame "ADC Reset ATF" {
      }
      frame "MCU Reset ATF" {
      }
      frame "Motor On ATF" {
        w407 = T2 [enum."Disabled and Grayed Out", enum."Disabled and Grayed Out", enum."Disabled and Grayed Out", enum."Disabled and Grayed Out", enum."Disabled and Grayed Out", enum."Enabled"] items=["Enabled", "Disabled", "Disabled and Grayed Out"] ("Disabled")
        n253 = Unbundle By Name(w415) -> ("Update drive ATF"=w414:refnum<vi>, "Gate driver ATF"=w413:refnum<vi>, "ADC reset ATF"=w412:refnum<vi>, "MCU reset ATF"=w411:refnum<vi>, "Motor On ATF"=w410:refnum<vi>, "Motor off ATF"=w409:refnum<vi>)
        n254 = Build Array(w414, w413, w412, w411, w410, w409) -> (w408:refnum<vi>[])
        n255 = call "enable disable.vi"("Disabled"=w407, "ref in"=w408) -> ()  [unwired: 10 in]
      }
      frame "Motor Off ATF" {
        w419 = T2 [enum."Enabled", enum."Enabled", enum."Enabled", enum."Enabled", enum."Enabled", enum."Disabled and Grayed Out"] items=["Enabled", "Disabled", "Disabled and Grayed Out"] ("Disabled")
        n256 = Unbundle By Name(w418) -> ("Update drive ATF"=w417:refnum<vi>, "Gate driver ATF"=w425:refnum<vi>, "ADC reset ATF"=w424:refnum<vi>, "MCU reset ATF"=w423:refnum<vi>, "Motor On ATF"=w422:refnum<vi>, "Motor off ATF"=w421:refnum<vi>)
        n257 = Build Array(w417, w425, w424, w423, w422, w421) -> (w420:refnum<vi>[])
        n258 = call "enable disable.vi"("Disabled"=w419, "ref in"=w420) -> ()  [unwired: 10 in]
      }
      frame "ADC Reset LOX" {
      }
      frame "MCU Reset LOX" {
      }
      frame "Gate Driver Power LOX" {
      }
      frame "Motor On LOX" {
        w433 = T2 [enum."Disabled and Grayed Out", enum."Disabled and Grayed Out", enum."Disabled and Grayed Out", enum."Disabled and Grayed Out", enum."Disabled and Grayed Out", enum."Enabled"] items=["Enabled", "Disabled", "Disabled and Grayed Out"] ("Disabled")
        n259 = Unbundle By Name(w441) -> ("Update drive lox"=w440:refnum<vi>, "Gate driver- LOX"=w439:refnum<vi>, "Adc reset lox"=w438:refnum<vi>, "MCU Reset -LOX"=w437:refnum<vi>, "Motor On lox"=w436:refnum<vi>, "Motor Off lox"=w435:refnum<vi>)
        n260 = Build Array(w440, w439, w438, w437, w436, w435) -> (w434:refnum<vi>[])
        n261 = call "enable disable.vi"("Disabled"=w433, "ref in"=w434) -> ()  [unwired: 10 in]
      }
      frame "Motor Off LOX" {
        w444 = T2 [enum."Enabled", enum."Enabled", enum."Enabled", enum."Enabled", enum."Enabled", enum."Disabled and Grayed Out"] items=["Enabled", "Disabled", "Disabled and Grayed Out"] ("Disabled")
        n262 = Unbundle By Name(w443) -> ("Update drive lox"=w451:refnum<vi>, "Gate driver- LOX"=w450:refnum<vi>, "Adc reset lox"=w449:refnum<vi>, "MCU Reset -LOX"=w448:refnum<vi>, "Motor On lox"=w447:refnum<vi>, "Motor Off lox"=w446:refnum<vi>)
        n263 = Build Array(w451, w450, w449, w448, w447, w446) -> (w445:refnum<vi>[])
        n264 = call "enable disable.vi"("Disabled"=w444, "ref in"=w445) -> ()  [unwired: 10 in]
      }
      frame "Connect PPSU" {
      }
      frame "DC ON PPSU" {
        w455 = T2 [enum."Disabled and Grayed Out", enum."Disabled and Grayed Out", enum."Disabled and Grayed Out", enum."Disabled and Grayed Out", enum."Enabled"] items=["Enabled", "Disabled", "Disabled and Grayed Out"] ("Disabled")
        n265 = Unbundle By Name(w462) -> ("update ppsu"=w461:refnum<vi>, "Alarm ack"=w460:refnum<vi>, "Ms initialize"=w459:refnum<vi>, "DC on"=w458:refnum<vi>, "DC off"=w457:refnum<vi>)
        n266 = Build Array(w461, w460, w459, w458, w457) -> (w456:refnum<vi>[])
        n267 = call "enable disable.vi"("Disabled"=w455, "ref in"=w456) -> ()  [unwired: 10 in]
      }
      frame "DC OFF PPSU" {
        w465 = T2 [enum."Enabled", enum."Enabled", enum."Enabled", enum."Enabled", enum."Disabled and Grayed Out"] items=["Enabled", "Disabled", "Disabled and Grayed Out"] ("Disabled")
        n268 = Unbundle By Name(w464) -> ("update ppsu"=w471:refnum<vi>, "Alarm ack"=w470:refnum<vi>, "Ms initialize"=w469:refnum<vi>, "DC on"=w468:refnum<vi>, "DC off"=w467:refnum<vi>)
        n269 = Build Array(w471, w470, w469, w468, w467) -> (w466:refnum<vi>[])
        n270 = call "enable disable.vi"("Disabled"=w465, "ref in"=w466) -> ()  [unwired: 10 in]
      }
      frame "Update PPSU Values" {
        n271 = flat-sequence {
          frame #0 {
          }
          frame #1 {
            n272 = One Button Dialog(message="The PPSU set parameters are updated.") -> ()  [unwired: 1 in, 1 out]
          }
        }
      }
      frame "Alarm Ack PPSU" {
      }
      frame "MS Initialize PPSU" {
      }
      frame "RT Exit" {
      }
      frame "Exit" {
        n273 = Unbundle By Name(w491) -> ("Data"=w490:refnum<notifier>)
        n274 = call "Enqueue Message.vi"("error in (no error)"=w486, "Message"="Exit", "Message Queue"=w484) -> ("error out"=w485:errorcluster)  [unwired: 7 in, 1 out]
        n275 = Release Queue(queue=w494, error in (no error)=w485) -> (error out=w489:errorcluster)  [unwired: 1 in, 2 out]
        n276 = Release Queue(queue=w484, error in (no error)=w489) -> (error out=w488:errorcluster)  [unwired: 1 in, 2 out]
        n277 = call "Fire User Event - Stop.vi"("error in (no error)"=w488, "User Event - Stop"=w495) -> ("error out"=w487:errorcluster)  [unwired: 9 in]
        n278 = Release Notifier(notifier=w490, error in (no error)=w487) -> (error out=w493:errorcluster)  [unwired: 1 in, 2 out]
        n279 = global write "Phase III Globals.vi" "Exit"(TRUE ("Exit")) -> ()
      }
      frame "Phase Code Name" {
        n280 = call "Phase code name.vi"("Enum"=enum16{"Read", "Write"}."Write", "error in"=w499, "Phase code W"="Datalog phase code") -> ("error out"=w498:errorcluster)  [unwired: 7 in, 1 out]
      }
      frame "Select Configuration" {
        n281 = call "Configuration File Name.vi"("Enum"=enum16{"Read", "Write"}."Write", "error in"=w504, "Phase code W"="CONFIGURATION FILE") -> ("error out"=w502:errorcluster)  [unwired: 7 in, 1 out]
      }
      frame "Daq Setting" {
        n282 = call "File & Folder.vi"("error in (no error)"=w519) -> ("error out"=w518:errorcluster, "File Output"=w517:T3)  [unwired: 9 in]
        n283 = Unbundle By Name(w517) -> ("Configuration path"=w509:path, "Sub vi's"=w516:path)
        n284 = Build Path(base path=w516, name or relative path=path "Hardware Config.vi") -> (appended path=w514:path)
        n285 = call "Call by reference.vi"("error in"=w518, "vi path"=w514) -> ("error out"=w510:errorcluster)  [unwired: 9 in]
        n286 = control-ref of="CONFIGURATION FILE"() -> (w511:refnum<vi>)
        n287 = List Folder(path=w509, error in=w510) -> (filenames=w508:string[], error out=w512:errorcluster)  [unwired: 2 in, 2 out]
        n288 = property class="CmbBox"(reference=w511, error in=w512, "Strings[]"=w508) -> (error out=w507:errorcluster)  [unwired: 1 out]
      }
      frame "Abort" {
      }
    }
    n289 = call "UI Error Handler - Message Handler.vi"("error in (no error)"=w98, "Message Queue"=w99) -> ()  [unwired: 9 in, 1 out]
    n290 = call <vilib>:"Clear Errors.vi"("error in (no error)"=w98) -> ("error out"=w109:errorcluster)  [unwired: 5 in, 1 out]
  }
  n291 = call "NS Reader.vi"("error in"=w8, "notifier in"=w9, "Message Queues in"=w10) -> ("error out"=w7:errorcluster)  [unwired: 7 in, 1 out]
  n292 = call "Queue Data log module.vi"("error in"=w8) -> ("error out"=w12:errorcluster)  [unwired: 10 in]
  n293 = while {
    tunnel: w25 -> [w530]
    tunnel: [w529] -> w24
    tunnel: w18 -> [w528]
    shift-right: [w526] -> w17
    shift-left: w8 -> [w527]
    stop <- w522 stop-if-true
    # "Event Loop"
    n294 = event shown="[35] \"Configure IP\": Value Change" {
      selector: w530 -> [_ _ _ _ _ _ _ _ _ _ _ _ _ _ _ _ _ _ _ _ _ _ _ _ _ _ _ _ _ _ _ _ _ _ _ _]
      dyn-events: [_ _ _ _ _ _ _ _ _ _ _ _ _ _ _ _ _ _ _ _ _ _ _ _ _ _ _ _ _ _ _ _ _ _ _ _] -> w529
      timeout: _ -> [_ _ _ _ _ _ _ _ _ _ _ _ _ _ _ _ _ _ _ _ _ _ _ _ _ _ _ _ _ _ _ _ _ _ _ _]
      tunnel: [_ _ _ _ TRUE _ _ _ _ _ _ _ _ _ _ _ _ _ _ _ _ _ _ _ _ _ _ _ _ _ _ _ _ _ _ _] -> w523
      tunnel: w528 -> [w538 w541 w549 w561 w567 w576 w580 w587 w590 w597 w603 w606 w613 w615 w620 w628 w630 w635 w640 w646 w652 w657 w662 w666 w673 w676 w682 w688 w694 w698 w703 w708 w713 w718 w723 w730]
      tunnel: w527 -> [w537 w543 w550 w563 w569 w575 w582 w584 w592 w596 w600 w608 w612 w618 w623 w626 w632 w638 w642 w648 w654 w660 w665 w669 w675 w679 w684 w690 w693 w700 w705 w710 w715 w720 w725 w729]
      tunnel: [w537 w542 w556 w562 w568 w574 w581 w585 w591 w595 w599 w607 w611 w617 w622 w625 w631 w637 w641 w647 w653 w659 w664 w668 w674 w678 w683 w689 w692 w699 w704 w709 w714 w719 w724 w728] -> w525
      tunnel: [w538 w539 w554 w559 w565 w573 w579 w586 w589 w594 w598 w605 w610 w616 w621 w627 w629 w636 w639 w645 w651 w658 w661 w667 w672 w677 w681 w687 w691 w697 w702 w707 w712 w717 w722 w727] -> w524
      event Timeout {
        n295 = event-data() -> ()  [unwired: 1 in, 3 out]
      }
      event "F_EPV_136", "F_EPV_131", "F_EPV_132", "F_EPV_21", "F_EPV_41", "N_EPV_68", "N_EPV_ 69", "N_EPV_ 33", "F_EPV_142", "F_EPV_28", "N_EPV_203", "N_EPV_206", "F_EPV_75", "C_EPV_2", "C_EPV_7", "C_EPV_8", "C_EPV_123", "C_EPV_127", "N_EPV_62a", "N_EPV_62b", "N_EPV_61", "G_EPV_51", "N_EPV_141", "C_EPV_803", "C_EPV_18", "C_EPV_1352", "N_EPV_202", "C_EPV_16": Value Change {
        n296 = event-data() -> ()  [unwired: 1 in, 1 out]
        n297 = call "Enqueue Message.vi"("error in (no error)"=w543, "Message"="Write DO", "Message Queue"=w541) -> ("error out"=w542:errorcluster, "dup Message Queue"=w539:refnum<queue>)  [unwired: 7 in]
      }
      event "START DAQ": Value Change {
        n298 = event-data() -> ()  [unwired: 1 in, 1 out]
        n299 = call "Enqueue Message.vi"("error in (no error)"=w550, "Message"="Update Configuration", "Message Queue"=w549) -> ("error out"=w547:errorcluster, "dup Message Queue"=w546:refnum<queue>)  [unwired: 7 in]
        n300 = call "Enqueue Message.vi"("error in (no error)"=w547, "Message"="Update Valve Statete Configuration", "Message Queue"=w546) -> ("error out"=w544:errorcluster, "dup Message Queue"=w545:refnum<queue>)  [unwired: 7 in]
        n301 = To Variant(anything=bool[] [TRUE, FALSE]) -> (Variant=w552:variant)
        n302 = call "Enqueue Message.vi"("error in (no error)"=w544, "Message Data"=w552, "Message"="Start Daq", "Message Queue"=w545) -> ("error out"=w556:errorcluster, "dup Message Queue"=w554:refnum<queue>)  [unwired: 6 in]
      }
      event "START LOG": Value Change {
        n303 = event-data() -> ()  [unwired: 1 in, 3 out]
        n304 = global write "Phase III Globals.vi" "Start Data log"(TRUE ("Start Daq")) -> ()
        n305 = global write "Phase III Globals.vi" "Stop Data log"(FALSE ("Start Daq")) -> ()
        n306 = call "Enqueue Message.vi"("error in (no error)"=w563, "Message"="Start Datalog", "Message Queue"=w561) -> ("error out"=w562:errorcluster, "dup Message Queue"=w559:refnum<queue>)  [unwired: 7 in]
      }
      event "EXIT": Value Change {
        n307 = event-data() -> ()  [unwired: 1 in, 1 out]
        n308 = call "Enqueue Message.vi"("Priority Message? (F)"=TRUE, "error in (no error)"=w569, "Message"="Exit", "Message Queue"=w567) -> ("error out"=w568:errorcluster, "dup Message Queue"=w565:refnum<queue>)  [unwired: 6 in]
      }
      event "STOP DAQ": Value Change {
        n309 = event-data() -> ()  [unwired: 1 in, 1 out]
        n310 = To Variant(anything=bool[] [FALSE, TRUE]) -> (Variant=w571:variant)
        n311 = call "Enqueue Message.vi"("error in (no error)"=w575, "Message Data"=w571, "Message"="Stop Daq", "Message Queue"=w576) -> ("error out"=w574:errorcluster, "dup Message Queue"=w573:refnum<queue>)  [unwired: 6 in]
      }
      event "Connect RT": Value Change {
        n312 = event-data() -> ()  [unwired: 1 in, 2 out]
        n313 = call "Enqueue Message.vi"("error in (no error)"=w582, "Message"="Connect RT", "Message Queue"=w580) -> ("error out"=w581:errorcluster, "dup Message Queue"=w579:refnum<queue>)  [unwired: 7 in]
      }
      event "Connect ppsu": Value Change {
        n314 = event-data() -> ()  [unwired: 1 in, 3 out]
        n315 = call "Enqueue Message.vi"("error in (no error)"=w584, "Message"="Connect PPSU", "Message Queue"=w587) -> ("error out"=w585:errorcluster, "dup Message Queue"=w586:refnum<queue>)  [unwired: 7 in]
      }
      event "DAQ SETTING": Value Change {
        n316 = event-data() -> ()  [unwired: 1 in, 1 out]
        n317 = call "Enqueue Message.vi"("error in (no error)"=w592, "Message"="Daq Setting", "Message Queue"=w590) -> ("error out"=w591:errorcluster, "dup Message Queue"=w589:refnum<queue>)  [unwired: 7 in]
      }
      event "HOLD UPDATE": Value Change {
        n318 = event-data() -> ()  [unwired: 1 in, 1 out]
        n319 = call "Enqueue Message.vi"("error in (no error)"=w596, "Message"="Hold Update", "Message Queue"=w597) -> ("error out"=w595:errorcluster, "dup Message Queue"=w594:refnum<queue>)  [unwired: 7 in]
      }
      event "IP ADDRESS": Value Change {
        n320 = event-data() -> ("NewVal"=w602:string)  [unwired: 1 in]
        n321 = call "Enqueue Message.vi"("error in (no error)"=w600, "Message Data"=w602, "Message"="Ip Config", "Message Queue"=w603) -> ("error out"=w599:errorcluster, "dup Message Queue"=w598:refnum<queue>)  [unwired: 6 in]
      }
      event "CONFIGURATION FILE": Value Change {
        n322 = event-data() -> ()  [unwired: 1 in, 1 out]
        n323 = call "Enqueue Message.vi"("error in (no error)"=w608, "Message"="Select Configuration", "Message Queue"=w606) -> ("error out"=w607:errorcluster, "dup Message Queue"=w605:refnum<queue>)  [unwired: 7 in]
      }
      event "ABORT": Value Change {
        n324 = event-data() -> ()  [unwired: 1 in, 1 out]
        n325 = call "Enqueue Message.vi"("error in (no error)"=w612, "Message"="Abort", "Message Queue"=w613) -> ("error out"=w611:errorcluster, "dup Message Queue"=w610:refnum<queue>)  [unwired: 7 in]
      }
      event "Datalog phase code": Value Change {
        n326 = event-data() -> ()  [unwired: 1 in, 6 out]
        n327 = call "Enqueue Message.vi"("error in (no error)"=w618, "Message"="Phase Code Name", "Message Queue"=w615) -> ("error out"=w617:errorcluster, "dup Message Queue"=w616:refnum<queue>)  [unwired: 7 in]
      }
      event "Connect Drive ATF": Value Change {
        n328 = event-data() -> ()  [unwired: 1 in, 6 out]
        n329 = call "Enqueue Message.vi"("error in (no error)"=w623, "Message"="Connect Drive ATF", "Message Queue"=w620) -> ("error out"=w622:errorcluster, "dup Message Queue"=w621:refnum<queue>)  [unwired: 7 in]
      }
      event "Connect Drive Lox": Value Change {
        n330 = event-data() -> ()  [unwired: 1 in, 1 out]
        n331 = call "Enqueue Message.vi"("error in (no error)"=w626, "Message"="Connect Drive LOX", "Message Queue"=w628) -> ("error out"=w625:errorcluster, "dup Message Queue"=w627:refnum<queue>)  [unwired: 7 in]
      }
      event "Alarm ack": Value Change {
        n332 = event-data() -> ()  [unwired: 1 in, 4 out]
        n333 = call "Enqueue Message.vi"("error in (no error)"=w632, "Message"="Alarm Ack PPSU", "Message Queue"=w630) -> ("error out"=w631:errorcluster, "dup Message Queue"=w629:refnum<queue>)  [unwired: 7 in]
      }
      event "Ms initialize": Value Change {
        n334 = event-data() -> ()  [unwired: 1 in, 4 out]
        n335 = call "Enqueue Message.vi"("error in (no error)"=w638, "Message"="MS Initialize PPSU", "Message Queue"=w635) -> ("error out"=w637:errorcluster, "dup Message Queue"=w636:refnum<queue>)  [unwired: 7 in]
      }
      event "update ppsu": Value Change {
        n336 = event-data() -> ()  [unwired: 1 in, 4 out]
        n337 = call "Enqueue Message.vi"("error in (no error)"=w642, "Message"="Update PPSU Values", "Message Queue"=w640) -> ("error out"=w641:errorcluster, "dup Message Queue"=w639:refnum<queue>)  [unwired: 7 in]
      }
      event "Update drive ATF": Value Change {
        n338 = event-data() -> ()  [unwired: 1 in, 4 out]
        n339 = call "Enqueue Message.vi"("error in (no error)"=w648, "Message"="Update Drive ATF Values", "Message Queue"=w646) -> ("error out"=w647:errorcluster, "dup Message Queue"=w645:refnum<queue>)  [unwired: 7 in]
      }
      event "STOP LOG": Value Change {
        n340 = event-data() -> ()  [unwired: 1 in, 4 out]
        n341 = global write "Phase III Globals.vi" "Start Data log"(FALSE ("Start Daq")) -> ()
        n342 = global write "Phase III Globals.vi" "Stop Data log"(TRUE ("Start Daq")) -> ()
        n343 = call "Enqueue Message.vi"("error in (no error)"=w654, "Message"="Stop Datalog", "Message Queue"=w652) -> ("error out"=w653:errorcluster, "dup Message Queue"=w651:refnum<queue>)  [unwired: 7 in]
      }
      event "Update drive lox": Value Change {
        n344 = event-data() -> ()  [unwired: 1 in, 4 out]
        n345 = call "Enqueue Message.vi"("error in (no error)"=w660, "Message"="Update Drive LOX Values", "Message Queue"=w657) -> ("error out"=w659:errorcluster, "dup Message Queue"=w658:refnum<queue>)  [unwired: 7 in]
      }
      event "Motor On lox": Value Change {
        n346 = event-data() -> ()  [unwired: 1 in, 4 out]
        n347 = call "Enqueue Message.vi"("error in (no error)"=w665, "Message"="Motor On LOX", "Message Queue"=w662) -> ("error out"=w664:errorcluster, "dup Message Queue"=w661:refnum<queue>)  [unwired: 7 in]
      }
      event "Motor Off lox": Value Change {
        n348 = event-data() -> ()  [unwired: 1 in, 4 out]
        n349 = call "Enqueue Message.vi"("error in (no error)"=w669, "Message"="Motor Off LOX", "Message Queue"=w666) -> ("error out"=w668:errorcluster, "dup Message Queue"=w667:refnum<queue>)  [unwired: 7 in]
      }
      event "DC on": Value Change {
        n350 = event-data() -> ()  [unwired: 1 in, 4 out]
        n351 = call "Enqueue Message.vi"("error in (no error)"=w675, "Message"="DC ON PPSU", "Message Queue"=w673) -> ("error out"=w674:errorcluster, "dup Message Queue"=w672:refnum<queue>)  [unwired: 7 in]
      }
      event "DC off": Value Change {
        n352 = event-data() -> ()  [unwired: 1 in, 4 out]
        n353 = call "Enqueue Message.vi"("error in (no error)"=w679, "Message"="DC OFF PPSU", "Message Queue"=w676) -> ("error out"=w678:errorcluster, "dup Message Queue"=w677:refnum<queue>)  [unwired: 7 in]
      }
      event "Gate driver- LOX": Value Change {
        n354 = event-data() -> ()  [unwired: 1 in, 4 out]
        n355 = call "Enqueue Message.vi"("error in (no error)"=w684, "Message"="Gate Driver Power LOX", "Message Queue"=w682) -> ("error out"=w683:errorcluster, "dup Message Queue"=w681:refnum<queue>)  [unwired: 7 in]
      }
      event "MCU Reset -LOX": Value Change {
        n356 = event-data() -> ()  [unwired: 1 in, 4 out]
        n357 = call "Enqueue Message.vi"("error in (no error)"=w690, "Message"="MCU Reset LOX", "Message Queue"=w688) -> ("error out"=w689:errorcluster, "dup Message Queue"=w687:refnum<queue>)  [unwired: 7 in]
      }
      event "Adc reset lox": Value Change {
        n358 = event-data() -> ()  [unwired: 1 in, 4 out]
        n359 = call "Enqueue Message.vi"("error in (no error)"=w693, "Message"="ADC Reset LOX", "Message Queue"=w694) -> ("error out"=w692:errorcluster, "dup Message Queue"=w691:refnum<queue>)  [unwired: 7 in]
      }
      event "Motor On ATF": Value Change {
        n360 = event-data() -> ()  [unwired: 1 in, 4 out]
        n361 = call "Enqueue Message.vi"("error in (no error)"=w700, "Message"="Motor On ATF", "Message Queue"=w698) -> ("error out"=w699:errorcluster, "dup Message Queue"=w697:refnum<queue>)  [unwired: 7 in]
      }
      event "Motor off ATF": Value Change {
        n362 = event-data() -> ()  [unwired: 1 in, 4 out]
        n363 = call "Enqueue Message.vi"("error in (no error)"=w705, "Message"="Motor Off ATF", "Message Queue"=w703) -> ("error out"=w704:errorcluster, "dup Message Queue"=w702:refnum<queue>)  [unwired: 7 in]
      }
      event "Gate driver ATF": Value Change {
        n364 = event-data() -> ()  [unwired: 1 in, 4 out]
        n365 = call "Enqueue Message.vi"("error in (no error)"=w710, "Message"="Gate Driver Power ATF", "Message Queue"=w708) -> ("error out"=w709:errorcluster, "dup Message Queue"=w707:refnum<queue>)  [unwired: 7 in]
      }
      event "MCU reset ATF": Value Change {
        n366 = event-data() -> ()  [unwired: 1 in, 4 out]
        n367 = call "Enqueue Message.vi"("error in (no error)"=w715, "Message"="MCU Reset ATF", "Message Queue"=w713) -> ("error out"=w714:errorcluster, "dup Message Queue"=w712:refnum<queue>)  [unwired: 7 in]
      }
      event "ADC reset ATF": Value Change {
        n368 = event-data() -> ()  [unwired: 1 in, 4 out]
        n369 = call "Enqueue Message.vi"("error in (no error)"=w720, "Message"="ADC Reset ATF", "Message Queue"=w718) -> ("error out"=w719:errorcluster, "dup Message Queue"=w717:refnum<queue>)  [unwired: 7 in]
      }
      event "Exit RT": Value Change {
        n370 = event-data() -> ()  [unwired: 1 in, 4 out]
        n371 = call "Enqueue Message.vi"("error in (no error)"=w725, "Message"="RT Exit", "Message Queue"=w723) -> ("error out"=w724:errorcluster, "dup Message Queue"=w722:refnum<queue>)  [unwired: 7 in]
      }
      event "Configure IP": Value Change {
        n372 = event-data() -> ()  [unwired: 1 in, 4 out]
        n373 = call "Enqueue Message.vi"("error in (no error)"=w729, "Message"="Ip Config", "Message Queue"=w730) -> ("error out"=w728:errorcluster, "dup Message Queue"=w727:refnum<queue>)  [unwired: 7 in]
      }
    }
    n374 = case shown="Error .." w525 {
      selector: w525 -> [w532 _]
      tunnel: [w532 _] -> w526
      tunnel: w524 -> [_ w535]
      tunnel: w523 -> [w531 _]
      tunnel: [w531 TRUE] -> w522
      frame No Error {
      }
      frame Error {
        n375 = call "Enqueue Message.vi"("Priority Message? (F)"=TRUE, "Message"="Exit", "Message Queue"=w535) -> ()  [unwired: 7 in, 2 out]
      }
    }
  }
  n376 = while {
    tunnel: w14 -> [w741]
    stop <- w736 stop-if-true
    # "Healths"
    # "Drive LOX"
    # "PPSU"
    # "DI Data"
    # "ATF Drive"
    # "Monitoring Loop"
    n377 = Get Date/Time In Seconds() -> (seconds since 1Jan1904=→"Time Stamp":timestamp)
    n378 = Wait on Notification(notifier=w741, timeout in ms (-1)=100) -> (error out=w737:errorcluster)  [unwired: 2 in, 3 out]
    n379 = Or(x=w737, y="EXIT") -> (x .or. y?=w736:bool)
    n380 = call "Log Health.vi"("Enum"=enum16{"Read", "Write"}."Read") -> ("Log health R"=→"LOG":bool)  [unwired: 9 in, 1 out]
    n381 = call "DI Search Channel.vi"() -> ("Array 2"=w732:bool[])  [unwired: 11 in]
    n382 = Index Array(array=w732) -> (element=→"F_EPV_136 HSS":bool)  [unwired: 1 in]
    n383 = Wait Until Next ms Multiple(millisecond multiple=u32 100) -> ()  [unwired: 1 out]
  }
  n384 = call "Destroy User Event - Stop.vi"("error in (no error)"=w13, "User Event - Stop"=w20) -> ("error out"=w21:errorcluster)  [unwired: 9 in]
  n385 = Unregister For Events(event registration refnum=w24, error in=w17) -> (error out=w23:errorcluster)
  n386 = Merge Errors(w12, w23, w21, w7) -> (w11:errorcluster)
  n387 = call <vilib>:"Simple Error Handler.vi"("error in (no error)"=w11) -> ()  [unwired: 4 in, 5 out]
